vi "MegaAwesome_10_10_12a_JW.vi"() -> ()   [LabVIEW 2011]
uses:
  data/MegaAwesome_States.ctl
  <vilib>/Utility/inputDevices.llb/keyboardAcquire.vi
  <vilib>/Utility/file.llb/Read From Spreadsheet File (string).vi
  <vilib>/Utility/file.llb/Write To Spreadsheet File (string).vi
panel:
  out "Save Next?":bool
  out "Image Center X":i32
  in  "Disable Flag":bool
  out "Index":string
  in  "Slider Min":dbl=5.0
  in  "Slider Max":dbl=5.0
  out "Opj X Axis":string
  out "X Axis Display Type":string
  in  "Index-Sat":dbl=5.0
  in  "Index-Lin":dbl=5.0
  in  "IndexLog-Lin":dbl=5.0
  in  "IndexLog-Sat":dbl=5.0 caption="Num Pts"
  out "Lin Id-Log Used":dbl[](array[numeric])
  out "Lin-Vg Array-Log Used":dbl[](array[numeric])
  in  "New: Comments":string
  out "Save Array":string[][](array[string])
  out "Folder Index":i32 caption="Length"
  out "Sat Id-Used":dbl[](array[numeric])
  out "Sat Vg Array-Used":dbl[](array[numeric])
  out "Vg Array-Log-Used":dbl[](array[numeric])
  out "Sat Id-Log-Used":dbl[](array[numeric])
  out "Lin Id-Used":dbl[](array[numeric])
  out "Lin-Vg Array-Used":dbl[](array[numeric])
  out "Lin Vd":dbl
  out "Recorded Prop":T1
  out "Current State":T2
  in  "Main Tab Control":T3(tab)
  in  "Transfer File":path
  out "Transfer Folder":path
  in  "Transport\nFolder":path caption="Transport Folder"
  out "Transport\nFile":path caption="Transport File"
  in  "Image Folder":path
  out "Image File":path
  out "Fabrication Prop":T4
  out "Distances":i32[](array[numeric])
  in  "Zoom":i32(slide)=-3 scale=-5.0..5.0
  in  "Magnification":i32(ring) items=["5x", "10x", "20x", "50x", "80x"]
  in  "Undo Button":bool
  in  "Remove Button":bool
  in  "Transfer Plots":T5(tab)=enum."Saturation"
  in  "Lin-Trans Slider":dbl(slide) step=1.0 scale=-40.0..40.0 scale format="%#_1p"
  out "Sqrt-Lin":cluster{dbl[], dbl[]}[](graph)
  in  "Sat-Trans Slider":dbl(slide) step=1.0 scale=-40.0..40.0 scale format="%#_1p"
  out "Sqrt-Sat":cluster{dbl[], dbl[]}[](graph)
  out "Raw- Lin":cluster{dbl[], dbl[]}[](graph)
  out "Raw- Sat":cluster{dbl[], dbl[]}[](graph)
  in  "Log Plots":enum32{"Linear", "Saturation", "Transport"}(tab)=enum."Saturation"
  in  "Lin-Log Slider":dbl(slide) step=1.0 scale=-40.0..40.0 scale format="%#_1p"
  out "Lin-Log":cluster{dbl[], dbl[]}[](graph)
  in  "Sat-Log Slider":dbl(slide) step=1.0 scale=-40.0..40.0 scale format="%#_1p"
  out "Sat-Log":cluster{dbl[], dbl[]}[](graph)
  out "Transport":cluster{ext[], ext[]}[](graph)
  out "Transport Name:":string
  in  "Manual Controls":T6
  in  "File Controls":T7
  out "Date Recorded":string="Date Recorded" caption="Measured"
  out "Data Name:":string
  out "Image Name":string
  out "Date Created":string caption="Fabricated"
  in  "Comments:":string
  out "Rec: Length":dbl caption="Length" format="%#_3g"
  out "Rec: Width":dbl caption="Width" format="%#_4g"
  out "Rec: Dielectric (d)":dbl caption="Dielectric (d)" format="%#_3g"
  in  "New: Dielectric":dbl
  in  "New: Length":dbl
  in  "New: Width":dbl
  out "Rec: Temp":dbl caption="Sample Temp" format="%.1f"
  in  "New: Temp":dbl format="%.1f"
  out "Image Out":T8(plugin-control)
  in  "Num Pts":dbl=5.0
  in  "Num Pts Log":dbl=5.0 caption="Num Pts"
  out "Recorded Values Cluster":T9
  out "Calculated Values Cluster":T9 caption="Recorded Values Cluster"
  out "Re-Calculated Values Cluster":T9 caption="Recorded Values Cluster"
  in  "Independant Variable:":string(combo)="Length (um):"
  out "Image Preview":T8(plugin-control)
  out "Total Width":i32
  in  "Index Array":i32(ring) caption="Index" items=["4C", "4C", "4C", "4C", "4C", "4C", "4C", "4C", "4C", "4C", "4C", "4C", "4C", "4C", "4C", "4C", "4C", "4C", "4C", "4C", "4C", "4C", "4C", "4C", "4C", "4C", "4C", "4C", "4C", "4C", "4C", "4C", "4C", "4C", "4C", "4C", "4C", "4C", "4C"]
  in  "Room Temp":dbl=294.0 caption="Room Temp (K)"
  out "No Image\n File":path=path "\\\\acad1\\physics/Jurchescu-group/JW-PD/Mega Awesome/Image Not Found.png" caption="No Image File"
  out "Origin Project File":path=path "\\\\acad1\\physics/Jurchescu-group/JW-PD/Group Library/Origin Project Files/DeviceData_8_10_12a_JW.opj"
  out "No Transport\n File":path=path "\\\\acad1\\physics/Jurchescu-group/JW-PD/Mega Awesome/No Transport File.txt" caption="No Transport File"
  in  "Transport Style Controls":T10={"Transport Line Size"=1, "Transport Line Color"=16772608} {"Transport Line Size" items=["Extra Small", "Small", "Medium", "Large", "Extra Large"]}
  out "Application Directory":path
  # "1)  Select the Transfer File that you would like to analyze:"
  # "Transfer Location"
  # "2) What else would you like to view during your analysis?"
  # "Transport Location"
  # "Image Location"
  # "Recorded"
  # "Calculated"
  # "Re-Calculated"
  # "Manual"
  # "um"
  # "Slider\nDoesn't\nWork"
  # "V"
  # "V"
  # "Slider\nDoesn't\nWork"
  # "V"
  # "Default File Choices"
  # "Default Analysis Values"
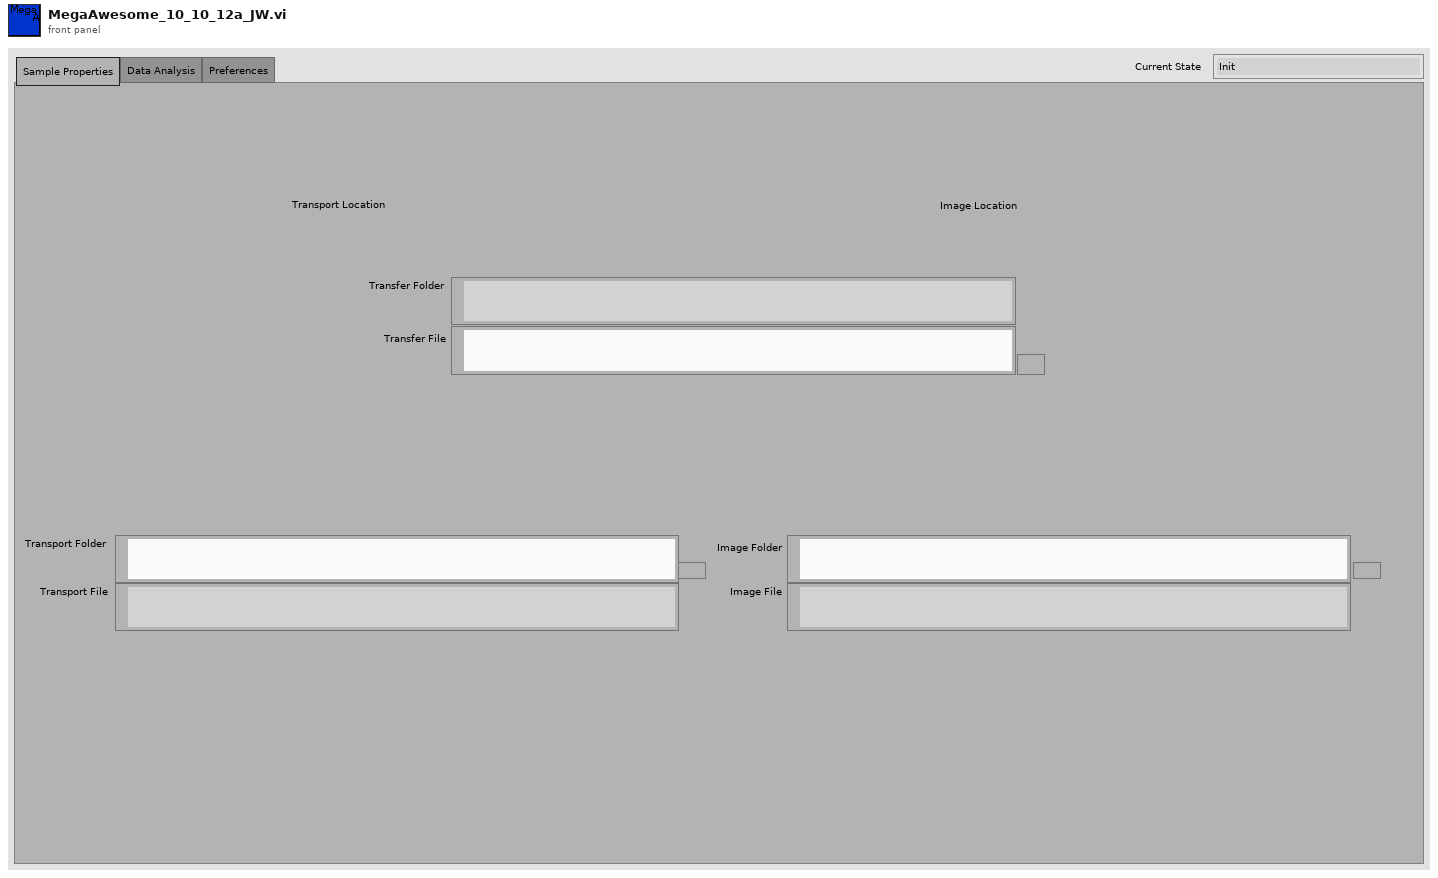
[diagram p1: front panel]
types:
  T1 = cluster{"Date Recorded":string, "Index":string, "Length":dbl, "Width":dbl, "Sample Temp":dbl}
  T2 = typedef "MegaAwesome_States.ctl" = enum16{"Init", "File Missing", "No Event", "Read Data", "Calculated Values", "Re-Calculated Values", "Next File", "Previous File", "Discard File", "Save", "Save Lines", "Export", "Exit"}
  T3 = enum32{"Sample Properties", "Data Analysis", "Preferences"}
  T4 = cluster{"Date Created":string, "Material":string, "Solvent":string, "Concentration":dbl, "Method":string, "Dielectric (nm)":dbl, "Treatment":string, "Comments":string}
  T5 = enum32{"Linear", "Saturation", "Raw-Linear", "Raw-Saturation"}
  T6 = cluster{"Manual-Temp":bool, "Manual-Width":bool, "Manuel-Length":bool, "Manuel-Dielectric":bool, "Manual Comments":bool}
  T7 = cluster{"Previous File":bool, "Discard ":bool, "Save Lines":bool, "Close":bool, "Next File ":bool, "Save":bool, "Save Next":bool, "Export":bool}
  T8 = typedef "IMAQ Image.ctl" = refnum<image>
  T9 = cluster{"Mobility-Sat":dbl, "Moblitity-Lin":dbl, "On/Off":dbl, "Off Current":dbl, "Vt-Sat":dbl, "STS":dbl, "Trap Density-VT":dbl, "Trap Density-STS":dbl}
  T10 = cluster{"Transport Line Size":u16, "Transport Line Color":u32}
  T11 = typedef "LVBoundsTypeDef.ctl" = cluster{"Width":u32, "Height":u32}
  T12 = enum16{"0", "1", "2", "3", "4", "5", "6", "7", "8", "9", "A", "B", "C", "D", "E", "F", "G", "H", "I", "J", "K", "L", "M", "N", "O", "P", "Q", "R", "S", "T", "U", "V", "W", "X", "Y", "Z", "F1", "F2", "F3", "F4", "F5", "F6", "F7", "F8", "F9", "F10", "F11", "F12", "F13", "F14", "F15", "ADD", "BACK", "BACKSLASH", "CAPITAL", "COMMA", "DECIMAL", "DELETE", "DIVIDE", "DOWN", "END", "EQUALS", "ESCAPE", "GRAVE (`)", "HOME", "INSERT", "LBRACKET", "LCONTROL", "LEFT", "L ALT", "LSHIFT", "LWIN", "MINUS", "MULTIPLY", "NEXT", "NUMLOCK", "NUMPAD_0", "NUMPAD_1", "NUMPAD_2", "NUMPAD_3", "NUMPAD_4", "NUMPAD_5", "NUMPAD_6", "NUMPAD_7", "NUMPAD_8", "NUMPAD_9", "PAUSE", "PERIOD", "PRIOR (PG UP)", "RBRACKET", "RCONTROL", "RETURN", "RIGHT", "R ALT", "RSHIFT", "RWIN", "SCROLL", "SEMICOLON", "SLASH", "SPACE", "SUBTRACT", "TAB", "UP", "ENTER (num pad)", "' (quote)"}[]
  T13 = enum16{"0", "1", "2", "3", "4", "5", "6", "7", "8", "9", "A", "B", "C", "D", "E", "F", "G", "H", "I", "J", "K", "L", "M", "N", "O", "P", "Q", "R", "S", "T", "U", "V", "W", "X", "Y", "Z", "F1", "F2", "F3", "F4", "F5", "F6", "F7", "F8", "F9", "F10", "F11", "F12", "F13", "F14", "F15", "ADD", "BACK", "BACKSLASH", "CAPITAL", "COMMA", "DECIMAL", "DELETE", "DIVIDE", "DOWN", "END", "EQUALS", "ESCAPE", "GRAVE (`)", "HOME", "INSERT", "LBRACKET", "LCONTROL", "LEFT", "L ALT", "LSHIFT", "LWIN", "MINUS", "MULTIPLY", "NEXT", "NUMLOCK", "NUMPAD_0", "NUMPAD_1", "NUMPAD_2", "NUMPAD_3", "NUMPAD_4", "NUMPAD_5", "NUMPAD_6", "NUMPAD_7", "NUMPAD_8", "NUMPAD_9", "PAUSE", "PERIOD", "PRIOR (PG UP)", "RBRACKET", "RCONTROL", "RETURN", "RIGHT", "R ALT", "RSHIFT", "RWIN", "SCROLL", "SEMICOLON", "SLASH", "SPACE", "SUBTRACT", "TAB", "UP", "ENTER (num pad)", "' (quote)"}
  T14 = typedef "ROI Descriptor" = cluster{"Global Rectangle":i32[], "Contours":cluster{"ID":enum32{"External", "Internal"}, "Type":u32, "Coordinates":i32[]}[]}
  T15 = cluster{string, dbl, bool, bool, bool, bool, bool, bool, i32}
  T16 = cluster{i32, cluster{string, dbl, bool, bool, bool, bool, bool, bool, i32}, i32, i32}
  T17 = cluster{"Global Rectangle":i32[], "Contours":cluster{"Contour Type":u32, "ROI Type":u32, "Points":i32[]}[]}
  T18 = cluster{"Contour Type":u32, "ROI Type":u32, "Points":i32[]}[]
  T19 = cluster{"[0]":cluster{dbl[], dbl[]}, "[1]":cluster{dbl[], dbl[]}, "[2]":cluster{dbl[], dbl[]}, "[3]":cluster{dbl[], dbl[]}, "[4]":cluster{dbl[], dbl[]}, "[5]":cluster{dbl[], dbl[]}, "[6]":cluster{dbl[], dbl[]}, "[7]":cluster{dbl[], dbl[]}, "[8]":cluster{dbl[], dbl[]}}
  T20 = cluster{i32[], cluster{"Contour Type":u32, "ROI Type":u32, "Points":i32[]}[]}
  T21 = cluster{"Contour Type":u32, "ROI Type":u32, "Points":i32[]}
  T22 = cluster{"Points[0]":i32, "Points[1]":i32, "Points[2]":i32, "Points[3]":i32, "Points[4]":i32, "Points[5]":i32, "Points[6]":i32, "Points[7]":i32, "Points[8]":i32}
  T23 = cluster{"Sat Vg Used":dbl[], "Sat Sqrt(Id) Used ":dbl[], "Lin Vg Used":dbl[], "Lin Sqrt(Id) Used":dbl[], "Index-Lin":dbl, "Index-Sat":dbl}
  T24 = cluster{"Raw Sat":cluster{dbl[], dbl[]}[], "Sqrt Sat":cluster{dbl[], dbl[]}[], "Log Sat":cluster{dbl[], dbl[]}[], "Raw Lin":cluster{dbl[], dbl[]}[], "Sqrt Lin":cluster{dbl[], dbl[]}[], "Log Lin":cluster{dbl[], dbl[]}[]}
  T25 = cluster{"Mobility-Sat":dbl, "Vt-Sat":dbl, "Mobility-Lin":dbl, "Vt-Lin":dbl, "Off I-Sat":dbl, "On/Off I-Sat":dbl}
  T26 = cluster{"Sat Vg Used":dbl[], "Sat Log(Id) Used":dbl[], "Lin Vg Used":dbl[], "Lin Log(Id) Used":dbl[], "STS Index-Sat":dbl, "STS Index-Lin":dbl}
  T27 = cluster{"Independant  Variable Indicator":string, "Parameter String Indicator":string}
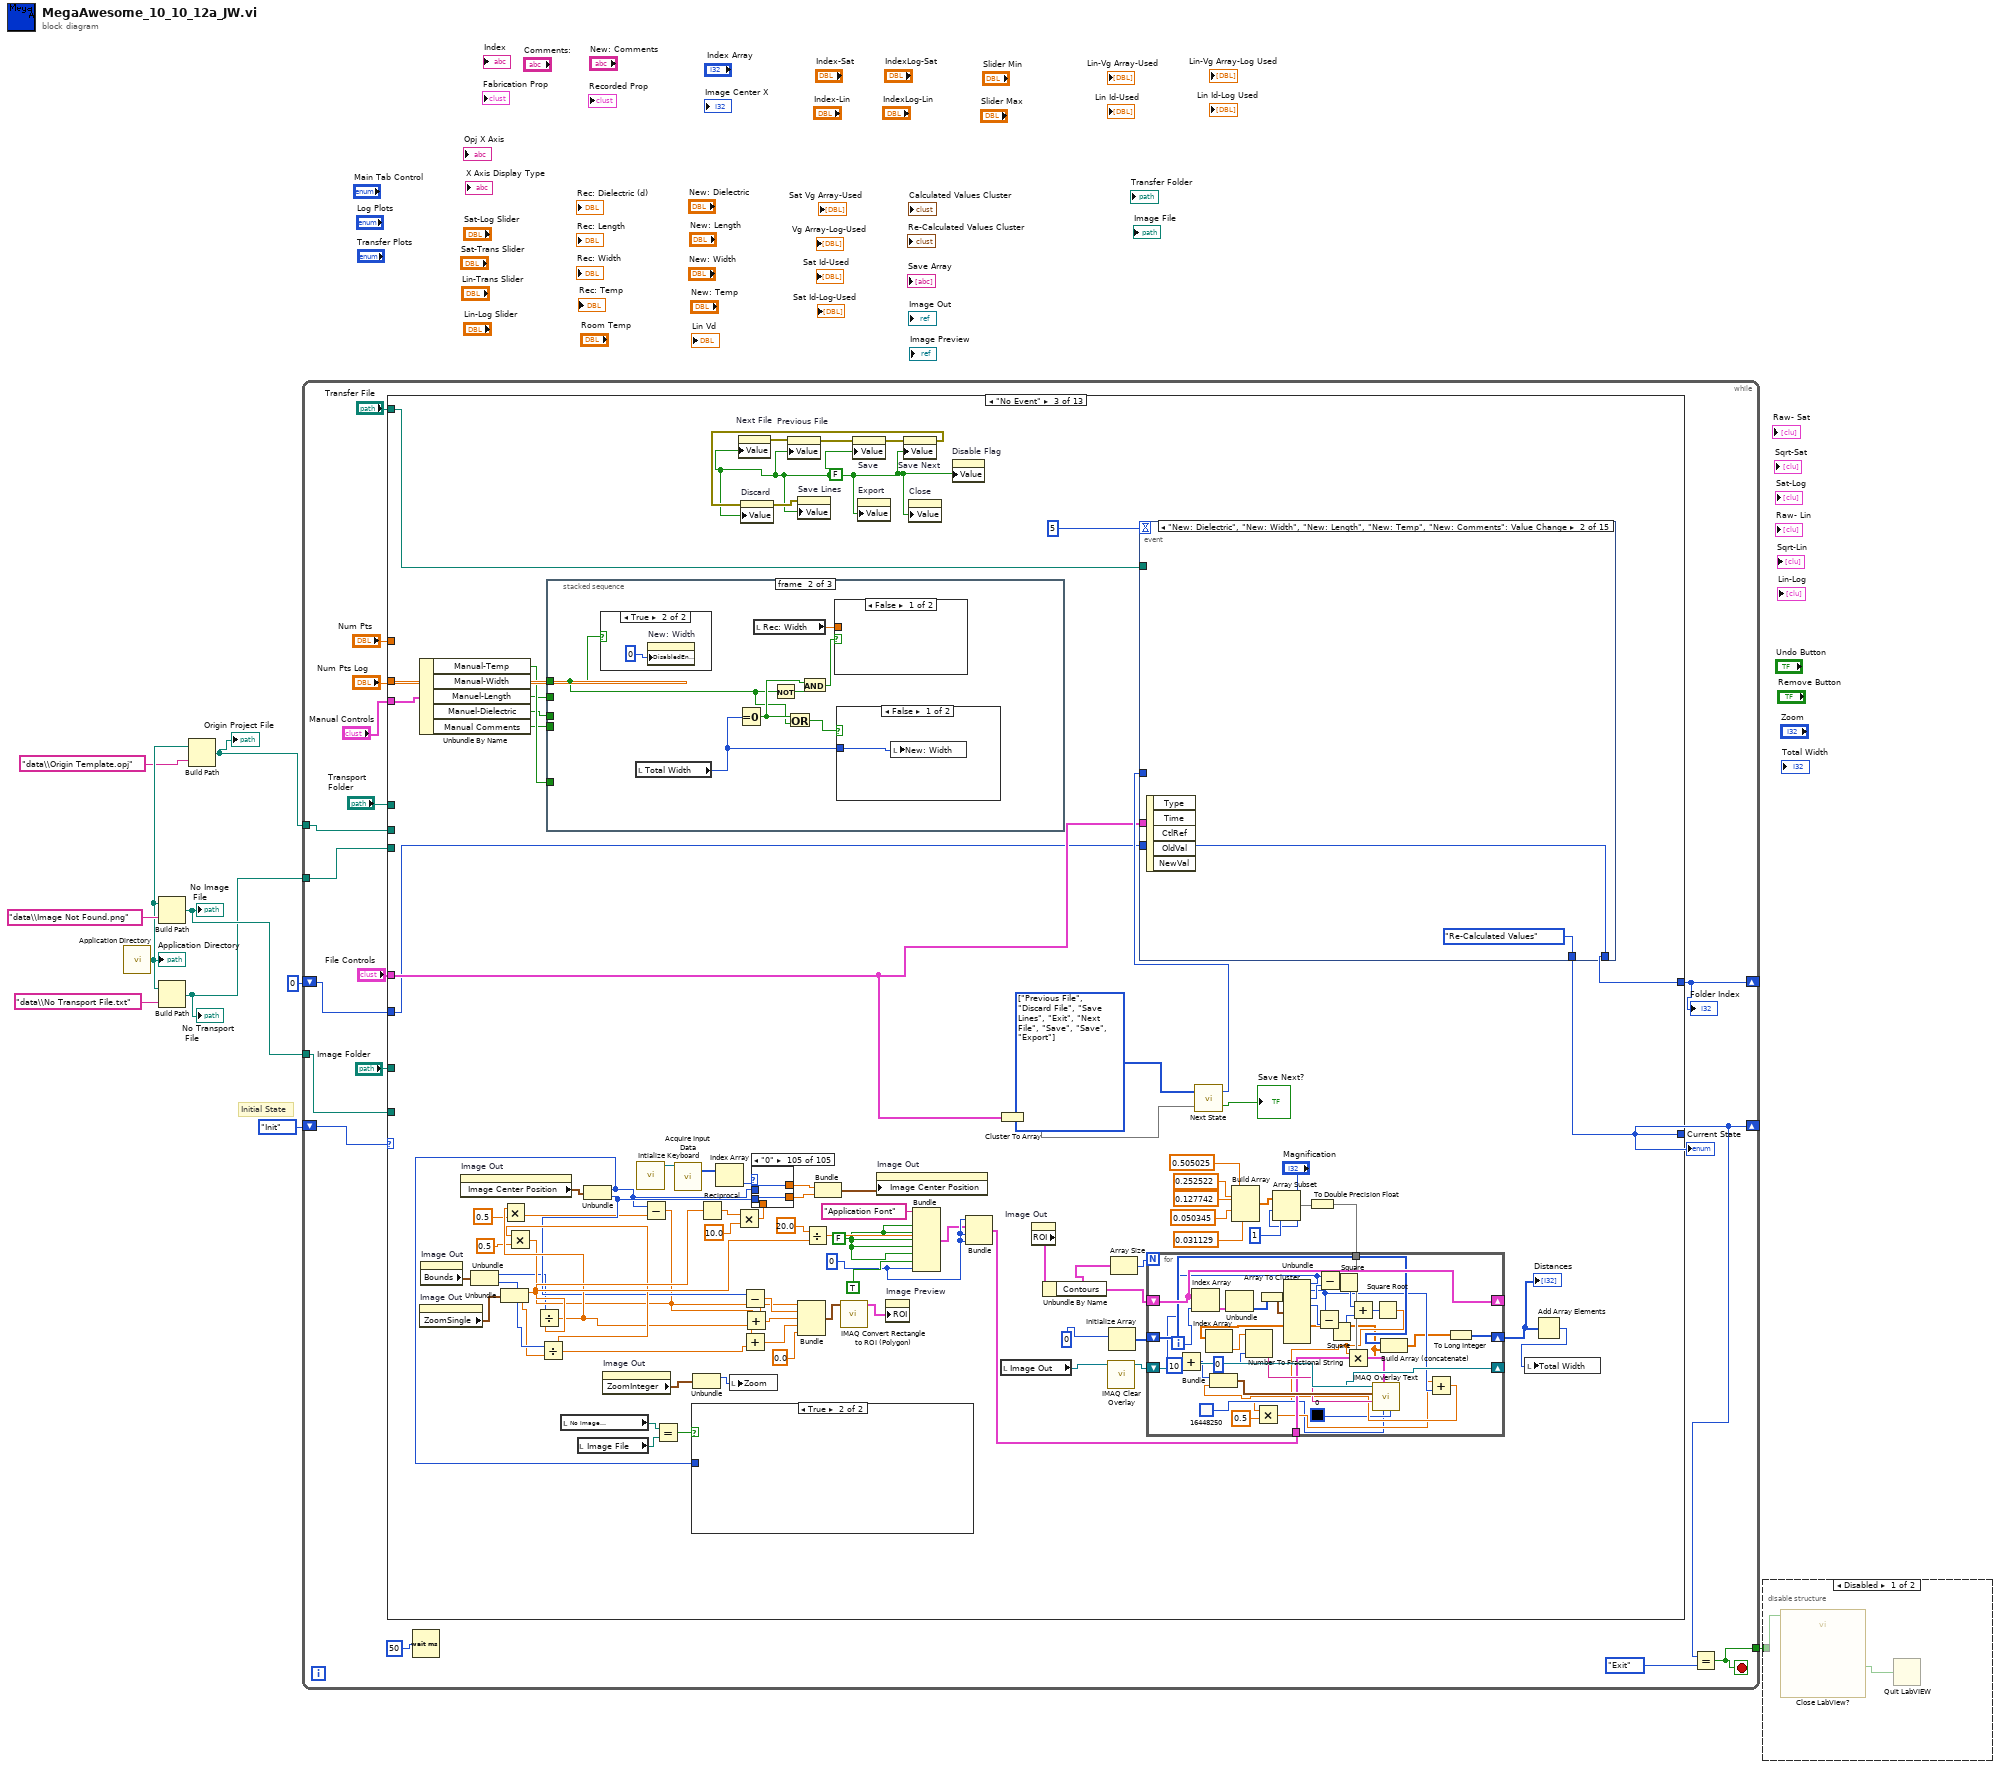
[diagram p0: block diagram]
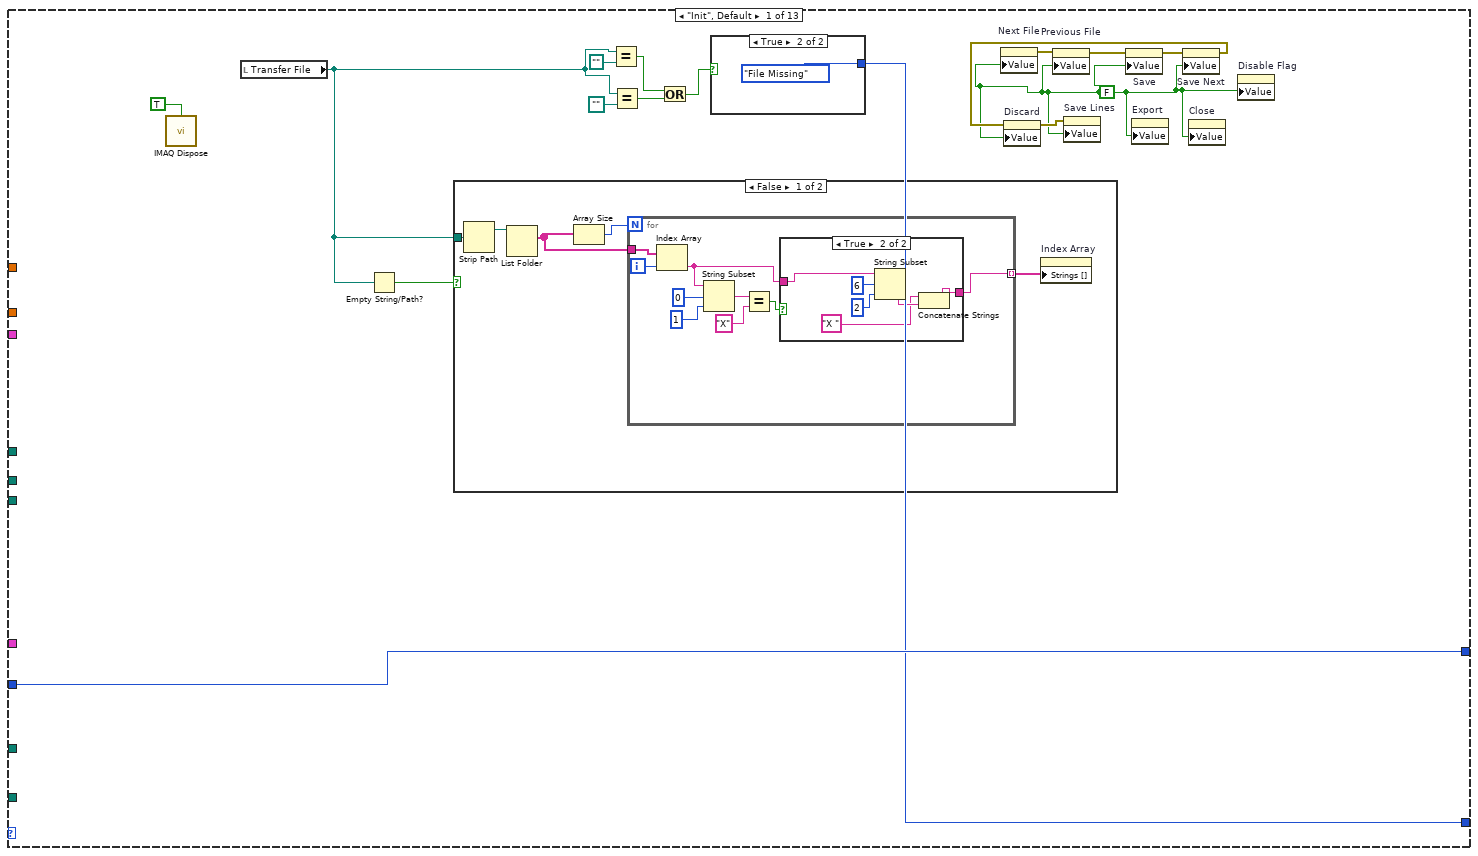
[diagram p3: hidden frame]
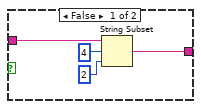
[diagram p4: hidden frame]
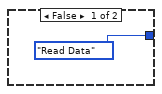
[diagram p6: hidden frame]
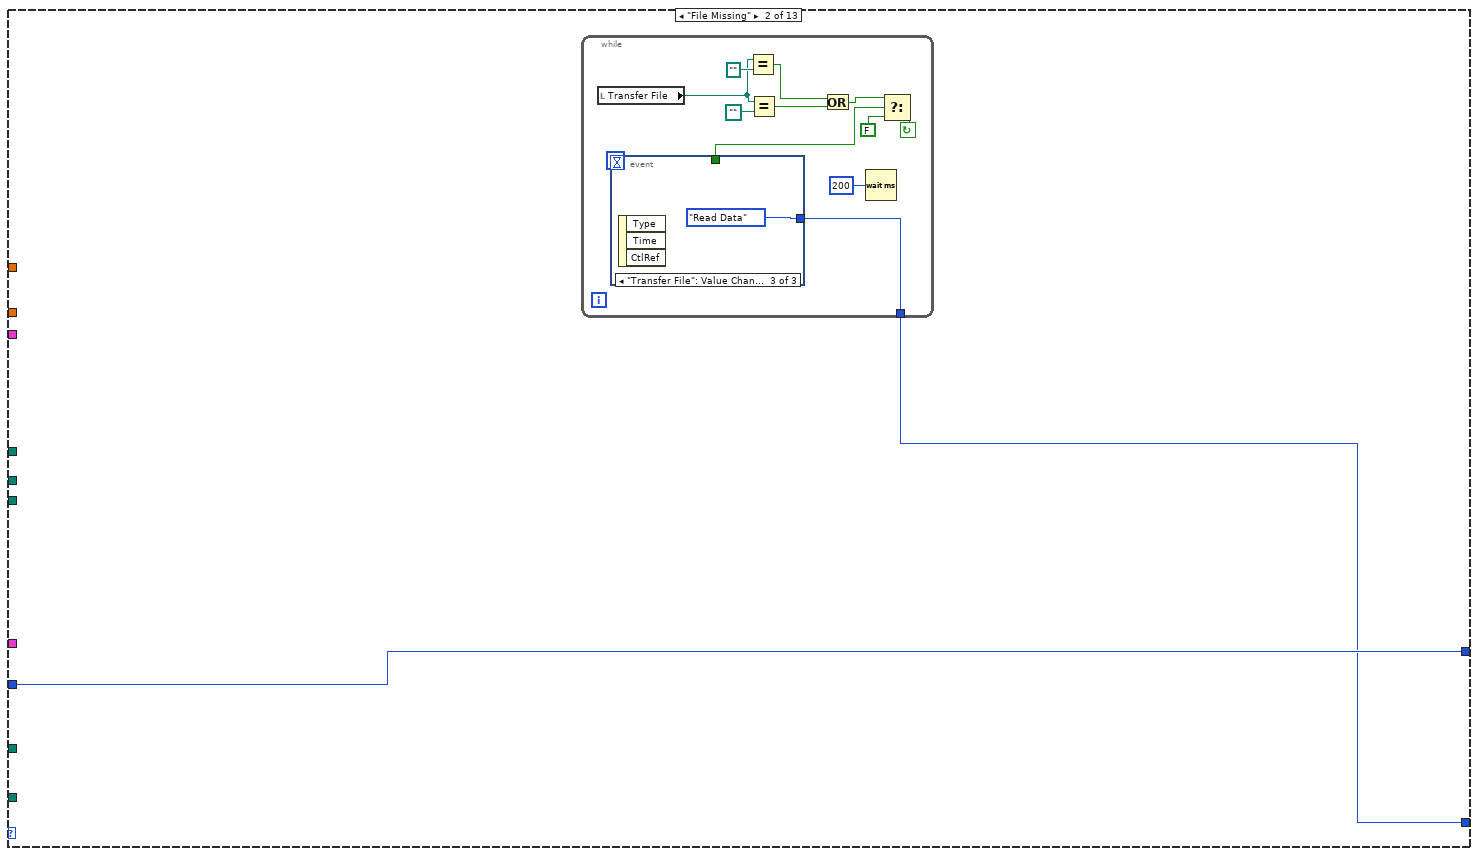
[diagram p7: hidden frame]
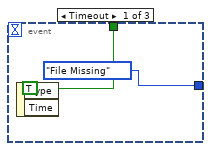
[diagram p8: hidden frame]
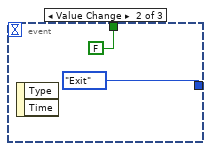
[diagram p9: hidden frame]
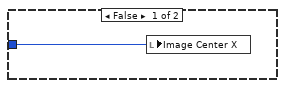
[diagram p10: hidden frame]
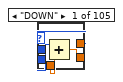
[diagram p11: hidden frame]
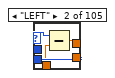
[diagram p12: hidden frame]
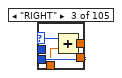
[diagram p13: hidden frame]
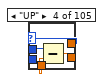
[diagram p14: hidden frame]
diagram:
  # "Initial State"
  n1 = call <vilib>:"Application Directory.vi"() -> ("Application Directory"=w3:path)
  "Application Directory" <- w3
  n2 = Build Path(base path=w3, name or relative path="data\\Image Not Found.png") -> (appended path=w6:path)
  "No Image\n File" <- w6
  n3 = Build Path(base path=w3, name or relative path="data\\No Transport File.txt") -> (appended path=w5:path)
  "No Transport\n File" <- w5
  n4 = Build Path(base path=w3, name or relative path="data\\Origin Template.opj") -> (appended path=w4:path)
  "Origin Project File" <- w4
  n5 = while {
    shift-right: [w11] -> _
    shift-left: MegaAwesome_States."Init" -> [w13]
    shift-right: [w21] -> _
    shift-left: 0 -> [w22]
    tunnel: w6 -> [w18]
    tunnel: w5 -> [w16]
    tunnel: w4 -> [w15]
    tunnel: [w14] -> w1
    stop <- w14 stop-if-true
    n6 = case shown="\"No Event\"" w13 {
      tunnel: [w28 w70 w164 MegaAwesome_States."Calculated Values" MegaAwesome_States."Re-Calculated Values" MegaAwesome_States."No Event" MegaAwesome_States."Read Data" MegaAwesome_States."Read Data" MegaAwesome_States."Init" w815 MegaAwesome_States."Exit" MegaAwesome_States."No Event" MegaAwesome_States."No Event"] -> w11
      tunnel: "Transfer File" -> [_ _ w156 w614 w662 _ w763 w774 w801 w820 _ _ _]
      tunnel: "Num Pts" -> [_ _ _ _ w697 _ _ _ _ _ _ _ _]
      tunnel: "Num Pts Log" -> [_ _ _ _ w696 _ _ _ _ _ _ _ _]
      tunnel: "Image Folder" -> [_ _ _ _ w693 _ _ _ _ _ _ w1350 _]
      tunnel: w18 -> [_ _ _ _ w692 _ _ _ _ _ _ _ _]
      tunnel: [w38 w71 w157 w619 w691 w723 w749 w772 w797 w821 w1336 w1360 w1366] -> w21
      tunnel: w22 -> [w38 w71 w89 w617 w691 w723 w750 w773 _ w821 w1336 w1360 w1366]
      tunnel: "Manual Controls" -> [_ _ w166 _ _ _ _ _ _ w819 _ _ _]
      tunnel: "File Controls" -> [_ _ w154 _ _ _ _ _ _ _ _ _ _]
      tunnel: "Transport\nFolder" -> [_ _ _ _ w658 _ _ _ _ _ _ _ _]
      tunnel: w16 -> [_ _ _ _ w657 _ _ _ _ _ _ _ _]
      tunnel: w15 -> [_ _ _ _ _ _ _ _ _ _ _ _ w1365]
      frame "Init", Default {
        w29 = FALSE
        n7 = call "IMAQ Dispose"("All Images? (No)"=TRUE) -> ()  [unwired: 5 in, 1 out]
        n8 = local read "Transfer File"() -> (w36:path)
        n9 = Empty String/Path?(string/path=w36) -> (empty?=w37:bool)
        n10 = case shown="False" w37 {
          tunnel: w36 -> [w45 _]
          frame False {
            n11 = Strip Path(path=w45) -> (stripped path=w47:path)  [unwired: 1 out]
            n12 = List Folder(path=w47) -> (filenames=w46:string[])  [unwired: 3 in, 3 out]
            n13 = Array Size(array=w46) -> (size(s)=w48:i32)
            n14 = for {
              N: w48 -> [_]
              tunnel: w46 -> [w57]
              tunnel: [w55] -> w44 mode=indexing
              i -> [w56]
              n15 = Index Array(array=w57, index=w56) -> (element=w54:string)
              n16 = String Subset(string=w54, offset (0)=0, length (rest)=1) -> (substring=w51:string)
              n17 = Equal?(x=w51, y="X") -> (x = y?=w50:bool)
              n18 = case shown="True" w50 {
                tunnel: w54 -> [w61 w65]
                tunnel: [w58 w64] -> w55
                frame False {
                  n19 = String Subset(string=w61, offset (0)=4, length (rest)=2) -> (substring=w58:string)
                }
                frame True {
                  n20 = String Subset(string=w65, offset (0)=6, length (rest)=2) -> (substring=w63:string)
                  n21 = Concatenate Strings("X ", w63) -> (w64:string)
                }
              }
            }
            n22 = property on="Index Array" class="Ring (strict)"("Strings []"=w44) -> ()  [unwired: 2 in, 2 out]
          }
          frame True {
          }
        }
        n23 = Equal?(x=w36, y=path "") -> (x = y?=w41:bool)
        n24 = Equal?(x=w36, y=path "") -> (x = y?=w40:bool)
        n25 = Or(x=w41, y=w40) -> (x .or. y?=w43:bool)
        n26 = case shown="True" w43 {
          tunnel: [MegaAwesome_States."Read Data" MegaAwesome_States."File Missing"] -> w28
          frame False {
          }
          frame True {
          }
        }
        n27 = property on="Next File" class="Bool (strict)"("Value"=w29) -> (error out=w34:errorcluster)  [unwired: 2 in, 1 out]
        n28 = property on="Previous File" class="Bool (strict)"(error in=w34, "Value"=w29) -> (error out=w33:errorcluster)  [unwired: 1 in, 1 out]
        n29 = property on="Save" class="Bool (strict)"(error in=w33, "Value"=w29) -> (error out=w32:errorcluster)  [unwired: 1 in, 1 out]
        n30 = property on="Export" class="Bool (strict)"("Value"=w29) -> ()  [unwired: 2 in, 2 out]
        n31 = property on="Save Next" class="Bool (strict)"(error in=w32, "Value"=w29) -> (error out=w31:errorcluster)  [unwired: 1 in, 1 out]
        n32 = property on="Discard" class="Bool (strict)"(error in=w31, "Value"=w29) -> (error out=w30:errorcluster)  [unwired: 1 in, 1 out]
        n33 = property on="Save Lines" class="Bool (strict)"(error in=w30, "Value"=w29) -> ()  [unwired: 1 in, 2 out]
        n34 = property on="Close" class="Bool (strict)"("Value"=w29) -> ()  [unwired: 2 in, 2 out]
        n35 = property on="Disable Flag" class="Bool (strict)"("Value"=w29) -> ()  [unwired: 2 in, 2 out]
      }
      frame "File Missing" {
        n36 = while {
          tunnel: [w78] -> w70
          stop <- w74 continue-if-true
          n37 = local read "Transfer File"() -> (w79:path)
          n38 = event shown="[2] \"Transfer File\": Value Change" {
            selector: _ -> [_ _ _]
            dyn-events: _ -> [_ _ _]
            timeout: 10 -> [_ _ _]
            tunnel: [MegaAwesome_States."File Missing" MegaAwesome_States."Exit" MegaAwesome_States."Read Data"] -> w78
            tunnel: [TRUE FALSE _] -> w77
            event Timeout {
              n39 = event-data() -> ()  [unwired: 1 in, 2 out]
            }
            event "File Controls.Close": Value Change {
              n40 = event-data() -> ()  [unwired: 1 in, 2 out]
            }
            event "Transfer File": Value Change {
              n41 = event-data() -> ()  [unwired: 1 in, 3 out]
            }
          }
          n42 = Equal?(x=w79, y=path "") -> (x = y?=w81:bool)
          n43 = Equal?(x=w79, y=path "") -> (x = y?=w82:bool)
          n44 = Or(x=w81, y=w82) -> (x .or. y?=w76:bool)
          n45 = Wait (ms)(milliseconds to wait=u32 200) -> ()  [unwired: 1 out]
          n46 = Select(t=w76, s=w77, f=FALSE) -> (s? t:f=w74:bool)
        }
      }
      frame "No Event" {
        w145 = FALSE
        w147 = 0
        w155 = FALSE
        w173 = T2[] [enum."Previous File", enum."Discard File", enum."Save Lines", enum."Exit", enum."Next File", enum."Save", enum."Save", enum."Export"] items=["Init", "File Missing", "No Event", "Read Data", "Calculated Values", "Re-Calculated Values", "Next File", "Previous File", "Discard File", "Save", "Save Lines", "Export", "Exit"]
        n47 = Unbundle By Name(w166) -> ("Manual-Temp"=w171:bool, "Manual-Width"=w170:bool, "Manuel-Length"=w169:bool, "Manuel-Dielectric"=w168:bool, "Manual Comments"=w167:bool)
        n48 = property on="Image Out" class="ImageControl"() -> ("ZoomSingle"=w131:cluster{"X":sgl, "Y":sgl})  [unwired: 2 in, 2 out]
        n49 = property on="Image Out" class="ImageControl"() -> ("Bounds"=w130:T11)  [unwired: 2 in, 2 out]
        n50 = property on="Image Out" class="ImageControl"() -> ("Image Center Position"=w124:cluster{"X":u32, "Y":u32})  [unwired: 2 in, 2 out]
        n51 = Unbundle(w130) -> ("Width"=w133:u32, "Height"=w134:u32)
        n52 = Unbundle(w131) -> ("X"=w151:sgl, "Y"=w132:sgl)
        n53 = Divide(x=w133, y=w151) -> (x/y=w142:sgl)
        n54 = Multiply(x=w142, y=0.5) -> (x*y=w137:dbl)
        n55 = Divide(x=w134, y=w132) -> (x/y=w143:sgl)
        n56 = Multiply(x=w143, y=0.5) -> (x*y=w138:dbl)
        n57 = stacked-sequence {
          tunnel: w171 -> [w573 _ _]
          tunnel: w170 -> [_ w582 _]
          tunnel: w169 -> [_ _ w598]
          tunnel: w168 -> [_ _ w595]
          tunnel: w167 -> [_ _ w594]
          frame #0 {
            n58 = local read "Rec: Temp"() -> (w572:dbl)
            n59 = case shown="False" w573 {
              tunnel: w572 -> [w578 _]
              frame False {
                n60 = local read "Rec: Temp"() -> (w576:dbl)
                n61 = property on="New: Temp" class="DigNum (strict)"("DisabledEnum"=1) -> ()  [unwired: 2 in, 2 out]
                n62 = Equal To 0?(x=w576) -> (x = 0?=w577:bool)
                n63 = local write "New: Temp"(w578) -> ()
                n64 = case shown="True" w577 {
                  tunnel: [w579 w580] -> w574
                  tunnel: w576 -> [w579 _]
                  frame False {
                  }
                  frame True {
                    n65 = local read "Room Temp"() -> (w580:dbl)
                  }
                }
                n66 = local write "Rec: Temp"(w574) -> ()
                n67 = local write "New: Temp"(w574) -> ()
              }
              frame True {
                n68 = property on="New: Temp" class="DigNum (strict)"("DisabledEnum"=0) -> ()  [unwired: 2 in, 2 out]
              }
            }
          }
          frame #1 {
            n69 = case shown="True" w582 {
              frame False {
                n70 = property on="New: Width" class="DigNum (strict)"("DisabledEnum"=1) -> ()  [unwired: 2 in, 2 out]
              }
              frame True {
                n71 = property on="New: Width" class="DigNum (strict)"("DisabledEnum"=0) -> ()  [unwired: 2 in, 2 out]
              }
            }
            n72 = local read "Total Width"() -> (w588:i32)
            n73 = Equal To 0?(x=w588) -> (x = 0?=w585:bool)
            n74 = local read "Rec: Width"() -> (w586:dbl)
            n75 = Not(x=w582) -> (.not. x?=w584:bool)
            n76 = Or(x=w585, y=w582) -> (x .or. y?=w587:bool)
            n77 = And(x=w585, y=w584) -> (x .and. y?=w583:bool)
            n78 = case shown="False" w583 {
              tunnel: w586 -> [_ w591]
              frame False {
              }
              frame True {
                n79 = local write "New: Width"(w591) -> ()
              }
            }
            n80 = case shown="False" w587 {
              tunnel: w588 -> [w592 _]
              frame False {
                n81 = local write "New: Width"(w592) -> ()
              }
              frame True {
                n82 = property on="New: Width" class="DigNum (strict)"("DisabledEnum"=0) -> ()  [unwired: 2 in, 2 out]
              }
            }
          }
          frame #2 {
            n83 = local read "Rec: Length"() -> (w599:dbl)
            n84 = case shown="False" w598 {
              tunnel: w599 -> [w607 _]
              frame False {
                n85 = local write "New: Length"(w607) -> ()
                n86 = property on="New: Length" class="DigNum (strict)"("DisabledEnum"=u8 1) -> ()  [unwired: 2 in, 2 out]
              }
              frame True {
                n87 = property on="New: Length" class="DigNum (strict)"("DisabledEnum"=0) -> ()  [unwired: 2 in, 2 out]
              }
            }
            n88 = local read "Comments:"() -> (w596:string)
            n89 = local read "Rec: Dielectric (d)"() -> (w597:dbl)
            n90 = case shown="False" w594 {
              tunnel: w596 -> [w601 _]
              frame False {
                n91 = local write "New: Comments"(w601) -> ()
                n92 = property on="New: Comments" class="Str"("DisabledEnum"=1) -> ()  [unwired: 2 in, 2 out]
              }
              frame True {
                n93 = property on="New: Comments" class="Str"("DisabledEnum"=0) -> ()  [unwired: 2 in, 2 out]
              }
            }
            n94 = case shown="True" w595 {
              tunnel: w597 -> [w604 _]
              frame False {
                n95 = local write "New: Dielectric"(w604) -> ()
                n96 = property on="New: Dielectric" class="DigNum (strict)"("DisabledEnum"=1) -> ()  [unwired: 2 in, 2 out]
              }
              frame True {
                n97 = property on="New: Dielectric" class="DigNum (strict)"("DisabledEnum"=0) -> ()  [unwired: 2 in, 2 out]
              }
            }
          }
        }
        n98 = local read "No Image\n File"() -> (w95:path)
        n99 = local read "Image File"() -> (w94:path)
        n100 = Unbundle(w124) -> ("X"=w96:u32, "Y"=w141:u32)
        n101 = property on="Image Out" class="ImageControl"() -> ("ZoomInteger"=w99:cluster{"X":i32, "Y":i32})  [unwired: 2 in, 2 out]
        n102 = call <vilib>:"Intialize Keyboard.vi"() -> ("device ID"=w121:refnum<k1>)  [unwired: 10 in, 1 out]
        n103 = Subtract(x=w96, y=w137) -> (x-y=w139:dbl)
        n104 = Equal?(x=w95, y=w94) -> (x = y?=w93:bool)
        n105 = call-poly <vilib>:"Acquire Input Data.vi"("device ID"=w121) -> ("keys pressed"=w122:T12)  [unwired: 16 in, 2 out]
        n106 = case shown="True" w93 {
          tunnel: w96 -> [w174 _]
          frame False {
            n107 = local write "Image Center X"(w174) -> ()
          }
          frame True {
          }
        }
        n108 = Unbundle(w99) -> ("X"=w98:i32)  [unwired: 1 out]
        n109 = Reciprocal(x=w151) -> (1/x=w152:sgl)
        n110 = Index Array(array=w122) -> (element=w118:T13)  [unwired: 1 in]
        n111 = local write "Zoom"(w98) -> ()
        n112 = Multiply(x=w152, y=sgl 10.0) -> (x*y=w150:sgl)
        n113 = property on="Next File" class="Bool (strict)"("Value"=w155) -> (error out=w162:errorcluster)  [unwired: 2 in, 1 out]
        n114 = Subtract(x=w141, y=w138) -> (x-y=w140:dbl)
        n115 = Add(x=w140, y=w143) -> (x+y=w126:dbl)
        n116 = Add(x=w139, y=w142) -> (x+y=w125:dbl)
        n117 = case shown="\"0\"" w118 {
          tunnel: w96 -> [w210 w216 w220 w222 w226 w228 w230 w232 w234 w236 w238 w240 w242 w244 w246 w248 w250 w252 w254 w256 w258 w260 w262 w264 w266 w268 w270 w272 w274 w276 w278 w280 w282 w284 w286 w288 w290 w292 w294 w296 w298 w300 w302 w304 w306 w308 w310 w312 w314 w316 w318 w320 w322 w324 w326 w328 w330 w332 w334 w336 w338 w340 w342 w344 w346 w348 w350 w352 w354 w356 w358 w360 w362 w364 w366 w368 w370 w372 w374 w376 w378 w380 w382 w384 w386 w388 w390 w392 w394 w396 w398 w400 w402 w404 w406 w408 w410 w412 w414 w416 w418 w420 w422 w424 w426]
          tunnel: [w210 w215 w219 w222 w226 w228 w230 w232 w234 w236 w238 w240 w242 w244 w246 w248 w250 w252 w254 w256 w258 w260 w262 w264 w266 w268 w270 w272 w274 w276 w278 w280 w282 w284 w286 w288 w290 w292 w294 w296 w298 w300 w302 w304 w306 w308 w310 w312 w314 w316 w318 w320 w322 w324 w326 w328 w330 w332 w334 w336 w338 w340 w342 w344 w346 w348 w350 w352 w354 w356 w358 w360 w362 w364 w366 w368 w370 w372 w374 w376 w378 w380 w382 w384 w386 w388 w390 w392 w394 w396 w398 w400 w402 w404 w406 w408 w410 w412 w414 w416 w418 w420 w422 w424 w426] -> w119
          tunnel: w141 -> [w212 w214 w218 w224 w225 w227 w229 w231 w233 w235 w237 w239 w241 w243 w245 w247 w249 w251 w253 w255 w257 w259 w261 w263 w265 w267 w269 w271 w273 w275 w277 w279 w281 w283 w285 w287 w289 w291 w293 w295 w297 w299 w301 w303 w305 w307 w309 w311 w313 w315 w317 w319 w321 w323 w325 w327 w329 w331 w333 w335 w337 w339 w341 w343 w345 w347 w349 w351 w353 w355 w357 w359 w361 w363 w365 w367 w369 w371 w373 w375 w377 w379 w381 w383 w385 w387 w389 w391 w393 w395 w397 w399 w401 w403 w405 w407 w409 w411 w413 w415 w417 w419 w421 w423 w425]
          tunnel: [w211 w214 w218 w223 w225 w227 w229 w231 w233 w235 w237 w239 w241 w243 w245 w247 w249 w251 w253 w255 w257 w259 w261 w263 w265 w267 w269 w271 w273 w275 w277 w279 w281 w283 w285 w287 w289 w291 w293 w295 w297 w299 w301 w303 w305 w307 w309 w311 w313 w315 w317 w319 w321 w323 w325 w327 w329 w331 w333 w335 w337 w339 w341 w343 w345 w347 w349 w351 w353 w355 w357 w359 w361 w363 w365 w367 w369 w371 w373 w375 w377 w379 w381 w383 w385 w387 w389 w391 w393 w395 w397 w399 w401 w403 w405 w407 w409 w411 w413 w415 w417 w419 w421 w423 w425] -> w120
          tunnel: w150 -> [w209 w213 w217 w221 _ _ _ _ _ _ _ _ _ _ _ _ _ _ _ _ _ _ _ _ _ _ _ _ _ _ _ _ _ _ _ _ _ _ _ _ _ _ _ _ _ _ _ _ _ _ _ _ _ _ _ _ _ _ _ _ _ _ _ _ _ _ _ _ _ _ _ _ _ _ _ _ _ _ _ _ _ _ _ _ _ _ _ _ _ _ _ _ _ _ _ _ _ _ _ _ _ _ _ _ _]
          frame "DOWN" {
            n118 = Add(x=w212, y=w209) -> (x+y=w211:sgl)
          }
          frame "LEFT" {
            n119 = Subtract(x=w216, y=w213) -> (x-y=w215:sgl)
          }
          frame "RIGHT" {
            n120 = Add(x=w220, y=w217) -> (x+y=w219:sgl)
          }
          frame "UP" {
            n121 = Subtract(x=w224, y=w221) -> (x-y=w223:sgl)
          }
          frame "ENTER (num pad)" {
          }
          frame "' (quote)" {
          }
          frame "END" {
          }
          frame "EQUALS" {
          }
          frame "ESCAPE" {
          }
          frame "GRAVE (`)" {
          }
          frame "HOME" {
          }
          frame "INSERT" {
          }
          frame "LBRACKET" {
          }
          frame "LCONTROL" {
          }
          frame "L ALT" {
          }
          frame "LSHIFT" {
          }
          frame "LWIN" {
          }
          frame "MINUS" {
          }
          frame "MULTIPLY" {
          }
          frame "NEXT" {
          }
          frame "NUMLOCK" {
          }
          frame "NUMPAD_0" {
          }
          frame "NUMPAD_1" {
          }
          frame "NUMPAD_2" {
          }
          frame "NUMPAD_3" {
          }
          frame "NUMPAD_4" {
          }
          frame "NUMPAD_5" {
          }
          frame "NUMPAD_6" {
          }
          frame "NUMPAD_7" {
          }
          frame "NUMPAD_8" {
          }
          frame "NUMPAD_9" {
          }
          frame "PAUSE" {
          }
          frame "PERIOD" {
          }
          frame "PRIOR (PG UP)" {
          }
          frame "RBRACKET" {
          }
          frame "RCONTROL" {
          }
          frame "RETURN" {
          }
          frame "R ALT" {
          }
          frame "RSHIFT" {
          }
          frame "RWIN" {
          }
          frame "SCROLL" {
          }
          frame "SEMICOLON" {
          }
          frame "SLASH" {
          }
          frame "SPACE" {
          }
          frame "SUBTRACT" {
          }
          frame "TAB" {
          }
          frame "DIVIDE" {
          }
          frame "DELETE" {
          }
          frame "DECIMAL" {
          }
          frame "COMMA" {
          }
          frame "CAPITAL" {
          }
          frame "BACKSLASH" {
          }
          frame "BACK" {
          }
          frame "ADD" {
          }
          frame "F15" {
          }
          frame "F14" {
          }
          frame "F13" {
          }
          frame "F12" {
          }
          frame "F11" {
          }
          frame "F10" {
          }
          frame "F9" {
          }
          frame "F8" {
          }
          frame "F7" {
          }
          frame "F6" {
          }
          frame "F5" {
          }
          frame "F4" {
          }
          frame "F3" {
          }
          frame "F2" {
          }
          frame "F1" {
          }
          frame "Z" {
          }
          frame "Y" {
          }
          frame "X" {
          }
          frame "W" {
          }
          frame "V" {
          }
          frame "U" {
          }
          frame "T" {
          }
          frame "S" {
          }
          frame "R" {
          }
          frame "Q" {
          }
          frame "P" {
          }
          frame "O" {
          }
          frame "N" {
          }
          frame "M" {
          }
          frame "L" {
          }
          frame "K" {
          }
          frame "J" {
          }
          frame "I" {
          }
          frame "H" {
          }
          frame "G" {
          }
          frame "F" {
          }
          frame "E" {
          }
          frame "D" {
          }
          frame "C" {
          }
          frame "B" {
          }
          frame "A" {
          }
          frame "9" {
          }
          frame "8" {
          }
          frame "7" {
          }
          frame "6" {
          }
          frame "5" {
          }
          frame "4" {
          }
          frame "3" {
          }
          frame "2" {
          }
          frame "1" {
          }
          frame "0" {
          }
        }
        n122 = property on="Previous File" class="Bool (strict)"(error in=w162, "Value"=w155) -> (error out=w161:errorcluster)  [unwired: 1 in, 1 out]
        n123 = Bundle(w139, w140, w125, w126, 0.0) -> (w127:cluster{dbl, dbl, dbl, dbl, dbl})  [unwired: 1 in]
        n124 = Divide(x=20.0, y=w151) -> (x/y=w149:dbl)
        n125 = Bundle("X"=w119, "Y"=w120) -> (w123:cluster{"X":sgl, "Y":sgl})  [unwired: 1 in]
        n126 = call "IMAQ Convert Rectangle to ROI (Polygon)"("Rectangle"=w127) -> ("ROI Descriptor"=w129:T14)  [unwired: 7 in, 2 out]
        n127 = property on="Save" class="Bool (strict)"(error in=w161, "Value"=w155) -> (error out=w160:errorcluster)  [unwired: 1 in, 1 out]
        n128 = property on="Export" class="Bool (strict)"("Value"=w155) -> ()  [unwired: 2 in, 2 out]
        n129 = property on="Image Out" class="ImageControl"("Image Center Position"=w123) -> ()  [unwired: 2 in, 2 out]
        n130 = property on="Image Preview" class="ImageControl"("ROI"=w129) -> ()  [unwired: 2 in, 2 out]
        n131 = property on="Save Next" class="Bool (strict)"(error in=w160, "Value"=w155) -> (error out=w159:errorcluster)  [unwired: 1 in, 1 out]
        n132 = property on="Discard" class="Bool (strict)"(error in=w159, "Value"=w155) -> (error out=w158:errorcluster)  [unwired: 1 in, 1 out]
        n133 = property on="Save Lines" class="Bool (strict)"(error in=w158, "Value"=w155) -> ()  [unwired: 1 in, 2 out]
        n134 = property on="Close" class="Bool (strict)"("Value"=w155) -> ()  [unwired: 2 in, 2 out]
        n135 = Bundle("Application Font", w149, w145, w145, w145, w145, w145, TRUE, w147) -> (w144:T15)  [unwired: 1 in]
        n136 = property on="Disable Flag" class="Bool (strict)"("Value"=w155) -> ()  [unwired: 2 in, 2 out]
        n137 = Bundle(w147, w144, w147, w147) -> (w101:T16)  [unwired: 1 in]
        n138 = Cluster To Array(cluster=w154) -> (array=w172:bool[])
        n139 = local read "Image Out"() -> (w100:T8)
        n140 = property on="Image Out" class="ImageControl"() -> ("ROI"=w103:T17)  [unwired: 2 in, 2 out]
        n141 = Unbundle By Name(w103) -> ("Contours"=w104:T18)
        n142 = call "IMAQ Clear Overlay"("Image"=w100) -> ("Image Out"=w117:T8)  [unwired: 9 in, 1 out]
        n143 = Initialize Array(0) -> (w106:i32[])  [unwired: 1 in]
        n144 = Array Size(array=w104) -> (size(s)=w105:i32)
        n145 = call "Next State.vi"("Buttons []"=w172, "States []"=w173) -> ("Save Next?"=→"Save Next?":bool, "Enum"=w165:T2)
        n146 = event shown="[1] \"New: Dielectric\", \"New: Width\", \"New: Length\", \"New: Temp\", \"New: Comments\": Value Change" {
          selector: _ -> [_ _ _ _ _ _ _ _ _ _ _ _ _ _ _]
          dyn-events: _ -> [_ _ _ _ _ _ _ _ _ _ _ _ _ _ _]
          timeout: 5 -> [_ _ _ _ _ _ _ _ _ _ _ _ _ _ _]
          tunnel: w165 -> [w428 _ _ _ _ _ _ _ _ _ _ _ _ _ _]
          tunnel: [w428 MegaAwesome_States."Re-Calculated Values" MegaAwesome_States."Calculated Values" MegaAwesome_States."Re-Calculated Values" MegaAwesome_States."Re-Calculated Values" MegaAwesome_States."Re-Calculated Values" MegaAwesome_States."Re-Calculated Values" MegaAwesome_States."Read Data" MegaAwesome_States."Read Data" MegaAwesome_States."No Event" MegaAwesome_States."No Event" MegaAwesome_States."No Event" MegaAwesome_States."No Event" MegaAwesome_States."No Event" MegaAwesome_States."No Event"] -> w164
          tunnel: w89 -> [w427 w429 w431 w433 w458 w486 w510 _ w538 w540 w553 w555 w559 w563 w567]
          tunnel: [w427 w429 w431 w433 w458 w486 w510 w529 w538 w540 w553 w555 w559 w563 w567] -> w157
          tunnel: w156 -> [_ _ _ _ _ _ _ w528 _ _ _ _ _ _ _]
          tunnel: w154 -> [_ _ _ _ _ _ _ _ _ _ _ _ _ _ _]
          event Timeout {
            n147 = event-data() -> ()  [unwired: 1 in, 2 out]
          }
          event "New: Dielectric", "New: Width", "New: Length", "New: Temp", "New: Comments": Value Change {
            n148 = event-data() -> ()  [unwired: 1 in, 5 out]
          }
          event "Num Pts Log", "Transport Style Controls", "Num Pts": Value Change {
            n149 = event-data() -> ()  [unwired: 1 in, 5 out]
          }
          event "Sat-Trans Slider": Value Change {
            n150 = event-data() -> ()  [unwired: 1 in, 5 out]
            n151 = local read "Sqrt-Sat"() -> (w457:cluster{dbl[], dbl[]}[])
            n152 = Decimate 1D Array(w457) -> (w441:cluster{dbl[], dbl[]}[], w442:cluster{dbl[], dbl[]}[])
            n153 = local read "Slider Min"() -> (w438:dbl)
            n154 = local read "Sat-Trans Slider"() -> (w436:dbl)
            n155 = Array To Cluster(array=w441) -> (cluster=w456:T19)
            n156 = local read "New: Dielectric"() -> (w451:dbl)
            n157 = local read "Num Pts"() -> (w434:dbl)
            n158 = local read "New: Width"() -> (w453:dbl)
            n159 = local read "New: Length"() -> (w452:dbl)
            n160 = Unbundle(w456) -> ("[0]"=w455:cluster{dbl[], dbl[]})  [unwired: 8 out]
            n161 = Absolute Value(x=w438) -> (abs(x)=w437:dbl)
            n162 = Unbundle(w455) -> (w439:dbl[], w454:dbl[])
            n163 = Add(x=w436, y=w437) -> (x+y=w435:dbl)
            n164 = Array Subset(array=w439, index=w435, length=w434) -> (w449:dbl[])
            n165 = local write "Sat Vg Array-Used"(w449) -> ()
            n166 = Array Subset(array=w454, index=w435, length=w434) -> (w450:dbl[])
            n167 = call "Mobility-Vt-Used Pts_Saturation.vi"("Width"=w453, "Length"=w452, "Dielectric (d)"=w451, "Sat Id Used"=w450, "Vg Used"=w449) -> ("Vt"=w445:dbl, "Mobility"=w446:dbl)  [unwired: 4 in, 1 out]
            n168 = local write "Index-Sat"(w435) -> ()
            n169 = local write "Sat Id-Used"(w450) -> ()
            n170 = Bundle(w449, w450) -> (w443:cluster{dbl[], dbl[]})  [unwired: 1 in]
            n171 = local read "Re-Calculated Values Cluster"() -> (w448:T9)
            n172 = Bundle By Name(cluster=w448, "Mobility-Sat"=w446, "Vt-Sat"=w445) -> (w447:T9)
            n173 = local write "Re-Calculated Values Cluster"(w447) -> ()
            n174 = Build Array (concatenate)(w441, w442, w443) -> (w440:cluster{dbl[], dbl[]}[])
            n175 = local write "Sqrt-Sat"(w440) -> ()
          }
          event "Lin-Trans Slider": Value Change {
            n176 = event-data() -> ()  [unwired: 1 in, 5 out]
            n177 = local read "Sqrt-Lin"() -> (w482:cluster{dbl[], dbl[]}[])
            n178 = Decimate 1D Array(w482) -> (w467:cluster{dbl[], dbl[]}[], w468:cluster{dbl[], dbl[]}[])
            n179 = local read "Slider Min"() -> (w464:dbl)
            n180 = Array To Cluster(array=w467) -> (cluster=w481:T19)
            n181 = local read "Lin-Trans Slider"() -> (w462:dbl)
            n182 = local read "New: Dielectric"() -> (w475:dbl)
            n183 = local read "Num Pts"() -> (w478:dbl)
            n184 = local read "New: Width"() -> (w477:dbl)
            n185 = local read "New: Length"() -> (w476:dbl)
            n186 = local read "Lin Vd"() -> (w459:dbl)
            n187 = Unbundle(w481) -> ("[0]"=w480:cluster{dbl[], dbl[]})  [unwired: 8 out]
            n188 = Absolute Value(x=w464) -> (abs(x)=w463:dbl)
            n189 = Unbundle(w480) -> (w465:dbl[], w479:dbl[])
            n190 = Add(x=w462, y=w463) -> (x+y=w461:dbl)
            n191 = Array Subset(array=w465, index=w461, length=w478) -> (w473:dbl[])
            n192 = local write "Lin-Vg Array-Used"(w473) -> ()
            n193 = Array Subset(array=w479, index=w461, length=w478) -> (w474:dbl[])
            n194 = call "Mobility-Vt-Used Pts_Linear.vi"("Width"=w477, "Length"=w476, "Vd"=w459, "Dielectric (d)"=w475, "Id Used"=w474, "Vg Used"=w473) -> ("Mobility"=w470:dbl)  [unwired: 3 in, 2 out]
            n195 = local write "Index-Lin"(w461) -> ()
            n196 = local write "Lin Id-Used"(w474) -> ()
            n197 = Bundle(w473, w474) -> (w469:cluster{dbl[], dbl[]})  [unwired: 1 in]
            n198 = local read "Re-Calculated Values Cluster"() -> (w472:T9)
            n199 = Bundle By Name(cluster=w472, "Moblitity-Lin"=w470) -> (w471:T9)
            n200 = local write "Re-Calculated Values Cluster"(w471) -> ()
            n201 = Build Array (concatenate)(w467, w468, w469) -> (w466:cluster{dbl[], dbl[]}[])
            n202 = local write "Sqrt-Lin"(w466) -> ()
          }
          event "Sat-Log Slider": Value Change {
            n203 = event-data() -> ()  [unwired: 1 in, 5 out]
            n204 = local read "Sat-Log"() -> (w489:cluster{dbl[], dbl[]}[])
            n205 = Decimate 1D Array(w489) -> (w496:cluster{dbl[], dbl[]}[], w497:cluster{dbl[], dbl[]}[])
            n206 = local read "Slider Min"() -> (w493:dbl)
            n207 = Array To Cluster(array=w496) -> (cluster=w506:T19)
            n208 = property on="Sat-Log" class="XYGraph (strict)"("Active Plot"=2, "Plot.Fill/Pt. Color"=u32 6618880, "Plot.Point Style"=11) -> ()  [unwired: 2 in, 2 out]
            n209 = local read "Num Pts Log"() -> (w503:dbl)
            n210 = local read "Sat-Log Slider"() -> (w491:dbl)
            n211 = Unbundle(w506) -> ("[0]"=w505:cluster{dbl[], dbl[]})  [unwired: 8 out]
            n212 = Absolute Value(x=w493) -> (abs(x)=w492:dbl)
            n213 = Unbundle(w505) -> (w494:dbl[], w504:dbl[])
            n214 = Add(x=w491, y=w492) -> (x+y=w488:dbl)
            n215 = Array Subset(array=w494, index=w488, length=w503) -> (w501:dbl[])
            n216 = Array Subset(array=w504, index=w488, length=w503) -> (w502:dbl[])
            n217 = local write "Vg Array-Log-Used"(w501) -> ()
            n218 = local write "IndexLog-Sat"(w488) -> ()
            n219 = Bundle(w501, w502) -> (w487:cluster{dbl[], dbl[]})  [unwired: 1 in]
            n220 = call "STS-Used.vi"("Id Used"=w502, "Vg-Used"=w501) -> ("STS"=w498:dbl)  [unwired: 9 in]
            n221 = local write "Sat Id-Log-Used"(w502) -> ()
            n222 = local read "Re-Calculated Values Cluster"() -> (w500:T9)
            n223 = Bundle By Name(cluster=w500, "STS"=w498) -> (w499:T9)
            n224 = local write "Re-Calculated Values Cluster"(w499) -> ()
            n225 = Build Array (concatenate)(w496, w497, w487) -> (w495:cluster{dbl[], dbl[]}[])
            n226 = local write "Sat-Log"(w495) -> ()
          }
          event "Lin-Log Slider": Value Change {
            n227 = event-data() -> ()  [unwired: 1 in, 5 out]
            n228 = local read "Lin-Log"() -> (w514:cluster{dbl[], dbl[]}[])
            n229 = Decimate 1D Array(w514) -> (w520:cluster{dbl[], dbl[]}[], w521:cluster{dbl[], dbl[]}[])
            n230 = local read "Slider Min"() -> (w517:dbl)
            n231 = Array To Cluster(array=w520) -> (cluster=w527:T19)
            n232 = local read "Num Pts Log"() -> (w524:dbl)
            n233 = property on="Lin-Log" class="XYGraph (strict)"("Active Plot"=2, "Plot.Fill/Pt. Color"=u32 6618880, "Plot.Point Style"=11) -> ()  [unwired: 2 in, 2 out]
            n234 = local read "Lin-Log Slider"() -> (w515:dbl)
            n235 = Unbundle(w527) -> ("[0]"=w526:cluster{dbl[], dbl[]})  [unwired: 8 out]
            n236 = Absolute Value(x=w517) -> (abs(x)=w516:dbl)
            n237 = Unbundle(w526) -> (w518:dbl[], w525:dbl[])
            n238 = Add(x=w515, y=w516) -> (x+y=w513:dbl)
            n239 = Array Subset(array=w518, index=w513, length=w524) -> (w522:dbl[])
            n240 = local write "Lin-Vg Array-Log Used"(w522) -> ()
            n241 = Array Subset(array=w525, index=w513, length=w524) -> (w523:dbl[])
            n242 = local write "IndexLog-Sat"(w513) -> ()
            n243 = Bundle(w522, w523) -> (w512:cluster{dbl[], dbl[]})  [unwired: 1 in]
            n244 = local write "Lin Id-Log Used"(w523) -> ()
            n245 = Build Array (concatenate)(w520, w521, w512) -> (w519:cluster{dbl[], dbl[]}[])
            n246 = local write "Lin-Log"(w519) -> ()
          }
          event "Index Array": Value Change {
            n247 = event-data() -> ()  [unwired: 1 in, 5 out]
            n248 = Strip Path(path=w528) -> (stripped path=w534:path)  [unwired: 1 out]
            n249 = local write "Transfer Folder"(w534) -> ()
            n250 = List Folder(path=w534) -> (filenames=w530:string[])  [unwired: 3 in, 3 out]
            n251 = local read "Index Array"() -> (w529:i32)
            n252 = Path To String(path=w534) -> (string=w535:string)
            n253 = Index Array(array=w530, index=w529) -> (element=w536:string)
            n254 = Concatenate Strings(w535, "\\", w536) -> (w532:string)
            n255 = String To Path(string=w532) -> (path=w531:path)
            n256 = local write "Transfer File"(w531) -> ()
          }
          event "Transfer File": Value Change {
            n257 = event-data() -> ()  [unwired: 1 in, 5 out]
          }
          event "Remove Button": Mouse Down {
            w542 = 0
            n258 = event-data() -> ()  [unwired: 1 in, 5 out]
            n259 = property on="Image Out" class="ImageControl"() -> ("ROI"=w552:T17)  [unwired: 2 in, 2 out]
            n260 = Unbundle(w552) -> ("Global Rectangle"=w543:i32[], "Contours"=w545:T18)
            n261 = Reverse 1D Array(array=w543) -> (reversed array=w544:i32[])
            n262 = Reverse 1D Array(array=w545) -> (reversed array=w546:T18)
            n263 = Delete From Array(array=w544, index=w542) -> (array with subset deleted=w547:i32[])  [unwired: 1 in, 1 out]
            n264 = Delete From Array(array=w546, index=w542) -> (array with subset deleted=w548:T18)  [unwired: 1 in, 1 out]
            n265 = Reverse 1D Array(array=w547) -> (reversed array=w549:i32[])
            n266 = Reverse 1D Array(array=w548) -> (reversed array=w550:T18)
            n267 = Bundle(w549, w550) -> (w551:T20)  [unwired: 1 in]
            n268 = property on="Image Out" class="ImageControl"("ROI"=w551) -> ()  [unwired: 2 in, 2 out]
          }
          event "Undo Button": Mouse Down {
            n269 = event-data() -> ()  [unwired: 1 in, 5 out]
            n270 = invoke on="Image Out" class="ImageControl" method="Clear ROI"() -> ()  [unwired: 3 in, 3 out]
          }
          event "Image Folder": Value Change {
            n271 = event-data() -> ()  [unwired: 1 in, 5 out]
            n272 = local read "Image File"() -> (w557:path)
            n273 = call "Vision Acquisition"("Image Path"=w557) -> ("Image Out"=w558:T8)  [unwired: 25 in, 1 out]
            n274 = local write "Image Preview"(w558) -> ()
            n275 = local write "Image Out"(w558) -> ()
          }
          event "Zoom": Value Change {
            n276 = event-data() -> ()  [unwired: 1 in, 5 out]
            n277 = local read "Zoom"() -> (w562:i32)
            n278 = Bundle("Zoom"=w562, "Zoom"=w562) -> (w561:cluster{"Zoom":i32, "Zoom":i32})  [unwired: 1 in]
            n279 = property on="Image Out" class="ImageControl"("ZoomInteger"=w561) -> ()  [unwired: 2 in, 2 out]
          }
          event "Image Out": Mouse Enter {
            n280 = event-data() -> ()  [unwired: 1 in, 3 out]
            n281 = call "Simulate_Keyboard.vi"("Action"=0, "Virtual Key"=162) -> ()  [unwired: 7 in, 1 out]
          }
          event "Image Out": Mouse Leave {
            n282 = event-data() -> ()  [unwired: 1 in, 3 out]
            n283 = flat-sequence {
              frame #0 {
                n284 = Wait (ms)(milliseconds to wait=10) -> ()  [unwired: 1 out]
              }
              frame #1 {
                n285 = call "Simulate_Keyboard.vi"("Action"=2, "Virtual Key"=162) -> ()  [unwired: 7 in, 1 out]
              }
            }
          }
        }
        n286 = Build Array(0.505025, 0.252522, 0.127742, 0.050345, 0.031129) -> (w113:dbl[])
        n287 = Array Subset(array=w113, index="Magnification", length=1) -> (w115:dbl[])
        n288 = To Double Precision Float(number=w115) -> (double precision float=w116:dbl[])
        n289 = for {
          N: w105 -> [_]
          shift-right: [w199] -> _
          shift-left: w104 -> [w199]
          shift-right: [w175] -> w91
          shift-left: w106 -> [w197]
          tunnel: w116 -> [w196]
          shift-right: [w193] -> _
          shift-left: w117 -> [w195]
          tunnel: w101 -> [w189]
          i -> [w192]
          n290 = Index Array(array=w199, index=w192) -> (element=w208:T21)
          n291 = Unbundle(w208) -> ("Points"=w207:i32[])  [unwired: 2 out]
          n292 = Array To Cluster(array=w207) -> (cluster=w206:T22)
          n293 = Unbundle(w206) -> ("Points[0]"=w188:i32, "Points[1]"=w185:i32, "Points[2]"=w198:i32, "Points[3]"=w204:i32)  [unwired: 5 out]
          n294 = Add(x=w188, y=10) -> (x+y=w186:i32)
          n295 = Subtract(x=w185, y=w204) -> (x-y=w203:i32)
          n296 = Subtract(x=w188, y=w198) -> (x-y=w205:i32)
          n297 = Square(x=w203) -> (x^2=w201:i32)
          n298 = Square(x=w205) -> (x^2=w202:i32)
          n299 = Add(x=w202, y=w201) -> (x+y=w200:i32)
          n300 = Square Root(x=w200) -> (sqrt(x)=w179:dbl)
          n301 = Multiply(x=w179, y=0.5) -> (x*y=w182:dbl)
          n302 = Multiply(x=w179, y=w196) -> (x*y=w178:dbl[])
          n303 = Index Array(array=w178) -> (element=w191:dbl)  [unwired: 1 in]
          n304 = Number To Fractional String(number=w191, precision (6)=0) -> (F-format string=w190:string)  [unwired: 2 in]
          n305 = Build Array (concatenate)(w197, w178) -> (w176:dbl[])
          n306 = Add(x=w182, y=w185) -> (x+y=w184:dbl)
          n307 = Bundle(w186, w184) -> (w194:cluster{i32, dbl})  [unwired: 1 in]
          n308 = call "IMAQ Overlay Text"("BG Color (Transparent)"=u32 0, "Text Color (black)"=u32 16448250, "Font, Size & Style"=w189, "String"=w190, "Origin"=w194, "Image"=w195) -> ("Image Out"=w193:T8)  [unwired: 4 in, 1 out]
          n309 = To Long Integer(number=w176) -> (32bit integer=w175:i32[])
        }
        "Distances" <- w91
        n310 = Add Array Elements(numeric array=w91) -> (sum=w102:i32)
        n311 = local write "Total Width"(w102) -> ()
      }
      frame "Read Data" {
        n312 = call "IMAQ Dispose"("All Images? (No)"=TRUE) -> ()  [unwired: 5 in, 1 out]
        n313 = case shown="True" "Disable Flag" {
          tunnel: w617 -> [_ w642]
          tunnel: [w638 w639] -> w616
          tunnel: w614 -> [w638 _]
          frame False {
          }
          frame True {
            n314 = local read "Transfer Folder"() -> (w641:path)
            n315 = List Folder(path=w641) -> (filenames=w643:string[])  [unwired: 3 in, 3 out]
            n316 = Index Array(array=w643, index=w642) -> (element=w640:string)
            n317 = Build Path(base path=w641, name or relative path=w640) -> (appended path=w639:path)
            n318 = local write "Transfer File"(w639) -> ()
          }
        }
        n319 = call "Recorded Values.vi"("Path"=w616) -> ("Recorded Char"=→"Recorded Values Cluster":T9, "Recorded Prop"=w629:T1, "Fabrication Prop"=w627:T4)  [unwired: 8 in]
        n320 = Strip Path(path=w616) -> (stripped path=w626:path, name=w625:string)
        n321 = local write "Fabrication Prop"(w627) -> ()
        n322 = local write "Recorded Prop"(w629) -> ()
        n323 = Unbundle By Name(w629) -> ("Date Recorded"=→"Date Recorded":string, "Index"=w628:string, "Length"=w622:dbl, "Width"=w621:dbl)  [unwired: 1 out]
        n324 = Unbundle By Name(w629) -> ("Sample Temp"=w631:dbl)
        n325 = Unbundle By Name(w627) -> ("Dielectric (nm)"=w623:dbl, "Comments"=w624:string, "Date Created"=→"Date Created":string)
        n326 = List Folder(path=w626) -> (filenames=w620:string[])  [unwired: 3 in, 3 out]
        n327 = local write "Rec: Dielectric (d)"(w623) -> ()
        n328 = local write "Index"(w628) -> ()
        n329 = local write "Rec: Length"(w622) -> ()
        n330 = local write "Rec: Width"(w621) -> ()
        n331 = Equal To 0?(x=w631) -> (x = 0?=w634:bool)
        n332 = Number To Decimal String(number=w631) -> (decimal integer string=w635:string)  [unwired: 1 in]
        n333 = local write "Comments:"(w624) -> ()
        n334 = Search 1D Array(1D array=w620, element=w625) -> (index of element=w619:i32)  [unwired: 1 in]
        n335 = Equal?(x="", y=w635) -> (x = y?=w633:bool)
        n336 = Index Array(array=w620, index=w619) -> (element=→"Data Name:":string)
        n337 = local write "New: Width"(w621) -> ()
        n338 = local write "New: Length"(w622) -> ()
        n339 = local write "Index Array"(w619) -> ()
        n340 = Or(x=w634, y=w633) -> (x .or. y?=w632:bool)
        n341 = local write "New: Dielectric"(w623) -> ()
        n342 = case shown="True" w632 {
          tunnel: [w644 w645] -> w613
          tunnel: w631 -> [w644 _]
          frame False {
          }
          frame True {
            n343 = local read "Room Temp"() -> (w645:dbl)
          }
        }
        n344 = local write "New: Temp"(w613) -> ()
        n345 = Bundle By Name(cluster=w629, "Sample Temp"=w613) -> (w630:T1)
        n346 = local write "Rec: Temp"(w613) -> ()
        n347 = local write "Recorded Prop"(w630) -> ()
      }
      frame "Calculated Values" {
        n348 = local read "Image Center X"() -> (w647:i32)
        n349 = call "Image from TRF Display.vi"("Image Center X"=w647, "No Image File"=w692, "Image Folder"=w693, "Transfer File"=w662) -> ("Image Preview"=w654:T8, "Image Out"=w655:T8, "Image File"=w656:path, "Image Name"=→"Image Name":string, "ROI File"=w651:path)  [unwired: 3 in]
        n350 = invoke on="Image Out" class="ImageControl" method="Clear ROI"() -> ()  [unwired: 3 in, 3 out]
        n351 = local write "Image File"(w656) -> ()
        n352 = local write "Image Out"(w655) -> ()
        n353 = local write "Image Preview"(w654) -> ()
        n354 = call <vilib>:"Check if File or Folder Exists.vi"("path"=w651) -> ("file or folder exists?"=w652:bool, "dup path"=w653:path)  [unwired: 8 in, 1 out]
        n355 = case shown="True" w652 {
          tunnel: w653 -> [_ w713]
          frame False {
          }
          frame True {
            n356 = Read from Text File(file (use dialog)=w713) -> (text=w717:string)  [unwired: 3 in, 3 out]
            n357 = property on="Image Out" class="ImageControl"() -> ("ROI"=w714:T17)  [unwired: 2 in, 2 out]
            n358 = Unflatten From String(type=w714, binary string=w717) -> (value=w715:T17, error out=w716:errorcluster)  [unwired: 3 in, 1 out]
            n359 = property on="Image Out" class="ImageControl"(error in=w716, "ROI"=w715) -> ()  [unwired: 1 in, 2 out]
          }
        }
        n360 = call "TRF to TSP Plot_09_21_12a_JW.vi"("Transport Graph Properties"="Transport Style Controls", "No Transport File"=w657, "Transport Folder"=w658, "Transfer File"=w662) -> ("Transport"=w663:cluster{ext[], ext[]}[], "Transport File"=→"Transport\nFile":path, "Transport Name"=→"Transport Name:":string)  [unwired: 5 in]
        "Transport" <- w663
        n361 = Array Size(array=w663) -> (size(s)=w661:i32)
        n362 = local read "Image Center X"() -> (w648:i32)
        n363 = for {
          N: w661 -> [_]
          tunnel: "Transport Style Controls" -> [w721]
          i -> [w720]
          n364 = Unbundle By Name(w721) -> ("Transport Line Size"=w718:u16, "Transport Line Color"=w719:u32)
          n365 = property on="Transport" class="XYGraph (strict)"("Active Plot"=w720, "Plot.Plot Color"=w719, "Plot.Line Width"=w718) -> ()  [unwired: 2 in, 2 out]
        }
        n366 = local read "Recorded Prop"() -> (w695:T1)
        n367 = local read "Fabrication Prop"() -> (w702:T4)
        n368 = Bundle("Image Center X"=w648, 0) -> (w650:cluster{"Image Center X":i32, i32})  [unwired: 1 in]
        n369 = property on="Image Out" class="ImageControl"("Image Center Position"=w650) -> ()  [unwired: 2 in, 2 out]
        n370 = local read "Calculated Values Cluster"() -> (w712:T9)
        n371 = call "Mobility-Vt Calculator-File.vi"("NumPts"=w697, "Path"=w662) -> ("Used Points"=w690:T23, "Graph Cluster"=w680:T24, "Lin Vd"=w665:dbl, "Output"=w710:T25)  [unwired: 6 in]
        n372 = call "STS Calculator-File.vi"("NumPts"=w696, "Path"=w662) -> ("Used Points"=w685:T26, "XY Graph-Sat"=w669:cluster{dbl[], dbl[]}[], "XY Graph-Lin"=w666:cluster{dbl[], dbl[]}[], "Ouput"=w705:cluster{"STS-Sat":dbl, "STS-Lin":dbl})  [unwired: 6 in]
        n373 = Unbundle By Name(w702) -> ("Dielectric (nm)"=w700:dbl)
        n374 = Unbundle By Name(w695) -> ("Sample Temp"=w694:dbl)
        n375 = Unbundle By Name(w710) -> ("Mobility-Sat"=w709:dbl, "Vt-Sat"=w701:dbl, "Mobility-Lin"=w708:dbl, "Off I-Sat"=w707:dbl, "On/Off I-Sat"=w706:dbl)  [unwired: 1 out]
        n376 = local write "Lin Vd"(w665) -> ()
        n377 = Unbundle By Name(w705) -> ("STS-Sat"=w699:dbl)  [unwired: 1 out]
        n378 = local write "Sat-Log"(w669) -> ()
        n379 = local write "Lin-Log"(w666) -> ()
        n380 = call "Trap Density_VT.vi"("VT"=w701, "Dielectric"=w700) -> ("Trap Density-VT"=w704:dbl)
        n381 = call "Trap Density_STS.vi"("Temp (T) [K]"=w694, "S.T.S. (S)"=w699, "Dielectric"=w700) -> ("Trap Density (N)"=w703:dbl)  [unwired: 8 in]
        n382 = Bundle By Name(cluster=w712, "Mobility-Sat"=w709, "Moblitity-Lin"=w708, "On/Off"=w706, "Off Current"=w707, "Vt-Sat"=w701, "STS"=w699, "Trap Density-VT"=w704, "Trap Density-STS"=w703) -> (w711:T9)
        n383 = Unbundle By Name(w685) -> ("Sat Vg Used"=w684:dbl[], "Sat Log(Id) Used"=w683:dbl[], "Lin Vg Used"=w682:dbl[], "Lin Log(Id) Used"=w681:dbl[], "STS Index-Sat"=w667:dbl, "STS Index-Lin"=w668:dbl)
        n384 = Unbundle By Name(w690) -> ("Sat Vg Used"=w689:dbl[], "Sat Sqrt(Id) Used"=w688:dbl[], "Lin Vg Used"=w687:dbl[], "Lin Sqrt(Id) Used"=w686:dbl[], "Index-Lin"=w676:dbl, "Index-Sat"=w675:dbl)
        n385 = local write "Vg Array-Log-Used"(w684) -> ()
        n386 = local write "Sat Id-Log-Used"(w683) -> ()
        n387 = local write "Lin-Vg Array-Log Used"(w682) -> ()
        n388 = local write "Lin Id-Log Used"(w681) -> ()
        n389 = local write "IndexLog-Sat"(w667) -> ()
        n390 = local write "Index-Lin"(w668) -> ()
        n391 = local write "Calculated Values Cluster"(w711) -> ()
        n392 = local write "Sat Vg Array-Used"(w689) -> ()
        n393 = local write "Sat Id-Used"(w688) -> ()
        n394 = local write "Lin-Vg Array-Used"(w687) -> ()
        n395 = local write "Lin Id-Used"(w686) -> ()
        n396 = local write "Index-Sat"(w675) -> ()
        n397 = local write "Index-Lin"(w676) -> ()
        n398 = local write "Lin-Log Slider"(w668) -> ()
        n399 = local write "Sat-Log Slider"(w667) -> ()
        n400 = local write "Sat-Trans Slider"(w675) -> ()
        n401 = local write "Lin-Trans Slider"(w676) -> ()
        n402 = Unbundle By Name(w680) -> ("Raw Sat"=w674:cluster{dbl[], dbl[]}[], "Sqrt Sat"=w677:cluster{dbl[], dbl[]}[], "Raw Lin"=w679:cluster{dbl[], dbl[]}[], "Sqrt Lin"=w678:cluster{dbl[], dbl[]}[])
        n403 = Index Array(array=w674) -> (element=w673:cluster{dbl[], dbl[]})  [unwired: 1 in]
        n404 = Unbundle(w673) -> (w672:dbl[])  [unwired: 1 out]
        n405 = Array Max & Min(array=w672) -> (max value=w671:dbl, min value=w670:dbl)  [unwired: 2 out]
        n406 = property on="Sat-Trans Slider" class="Slide (strict)"("Scale.Maximum"=w671, "Scale.Minimum"=w670) -> ()  [unwired: 2 in, 2 out]
        n407 = property on="Lin-Trans Slider" class="Slide (strict)"("Scale.Maximum"=w671, "Scale.Minimum"=w670) -> ()  [unwired: 2 in, 2 out]
        n408 = property on="Sat-Log Slider" class="Slide (strict)"("Scale.Maximum"=w671, "Scale.Minimum"=w670) -> ()  [unwired: 2 in, 2 out]
        n409 = property on="Lin-Log Slider" class="Slide (strict)"("Scale.Maximum"=w671, "Scale.Minimum"=w670) -> ()  [unwired: 2 in, 2 out]
        n410 = local write "Slider Max"(w671) -> ()
        n411 = local write "Slider Min"(w670) -> ()
        n412 = local write "Raw- Sat"(w674) -> ()
        n413 = local write "Raw- Lin"(w679) -> ()
        n414 = local write "Sqrt-Sat"(w677) -> ()
        n415 = local write "Sqrt-Lin"(w678) -> ()
      }
      frame "Re-Calculated Values" {
        n416 = local read "Vg Array-Log-Used"() -> (w730:dbl[])
        n417 = local read "Sat Vg Array-Used"() -> (w738:dbl[])
        n418 = local read "Lin-Vg Array-Used"() -> (w744:dbl[])
        n419 = local read "Sat Id-Log-Used"() -> (w729:dbl[])
        n420 = local read "New: Dielectric"() -> (w742:dbl)
        n421 = local read "New: Dielectric"() -> (w727:dbl)
        n422 = local read "New: Length"() -> (w741:dbl)
        n423 = local read "New: Length"() -> (w737:dbl)
        n424 = local read "New: Width"() -> (w740:dbl)
        n425 = local read "New: Width"() -> (w736:dbl)
        n426 = local read "Lin Id-Used"() -> (w743:dbl[])
        n427 = local read "Sat Id-Used"() -> (w735:dbl[])
        n428 = local read "Re-Calculated Values Cluster"() -> (w746:T9)
        n429 = local read "New: Dielectric"() -> (w726:dbl)
        n430 = local read "New: Temp"() -> (w725:dbl)
        n431 = local read "Lin Vd"() -> (w722:dbl)
        n432 = call "Mobility-Vt-Used Pts_Saturation.vi"("Width"=w736, "Length"=w737, "Dielectric (d)"=w727, "Sat Id Used"=w735, "Vg Used"=w738) -> ("Vt"=w733:dbl, "Mobility"=w734:dbl)  [unwired: 4 in, 1 out]
        n433 = call "STS-Used.vi"("Id Used"=w729, "Vg-Used"=w730) -> ("STS"=w728:dbl)  [unwired: 9 in]
        n434 = call "Mobility-Vt-Used Pts_Linear.vi"("Width"=w740, "Length"=w741, "Vd"=w722, "Dielectric (d)"=w742, "Id Used"=w743, "Vg Used"=w744) -> ("Mobility"=w739:dbl)  [unwired: 3 in, 2 out]
        n435 = call "Trap Density_VT.vi"("VT"=w733, "Dielectric"=w727) -> ("Trap Density-VT"=w732:dbl)
        n436 = call "Trap Density_STS.vi"("Temp (T) [K]"=w725, "S.T.S. (S)"=w728, "Dielectric"=w726) -> ("Trap Density (N)"=w724:dbl)  [unwired: 8 in]
        n437 = Bundle By Name(cluster=w746, "Mobility-Sat"=w734, "Moblitity-Lin"=w739, "Vt-Sat"=w733, "STS"=w728, "Trap Density-VT"=w732, "Trap Density-STS"=w724) -> (w745:T9)
        n438 = local write "Re-Calculated Values Cluster"(w745) -> ()
      }
      frame "Next File" {
        n439 = call "IMAQ Dispose"("All Images? (No)"=TRUE) -> ()  [unwired: 5 in, 1 out]
        n440 = Strip Path(path=w763) -> (stripped path=w754:path, name=w761:string)
        n441 = local write "Transfer Folder"(w754) -> ()
        n442 = List Folder(path=w754) -> (filenames=w748:string[])  [unwired: 3 in, 3 out]
        n443 = Array Size(array=w748) -> (size(s)=w760:i32)
        n444 = Search 1D Array(1D array=w748, element=w761) -> (index of element=w758:i32)  [unwired: 1 in]
        n445 = Decrement(x=w760) -> (x-1=w759:i32)
        n446 = Equal?(x=w759, y=w758) -> (x = y?=w757:bool)
        n447 = case shown="True" w757 {
          tunnel: w750 -> [w765 _]
          tunnel: [w764 0] -> w749
          frame False {
            n448 = Increment(x=w765) -> (x+1=w764:i32)
          }
          frame True {
          }
        }
        n449 = Path To String(path=w754) -> (string=w755:string)
        n450 = Index Array(array=w748, index=w749) -> (element=w756:string)
        n451 = Concatenate Strings(w755, "\\", w756) -> (w752:string)
        n452 = String To Path(string=w752) -> (path=w751:path)
        n453 = local write "Transfer File"(w751) -> ()
      }
      frame "Previous File" {
        n454 = call "IMAQ Dispose"("All Images? (No)"=TRUE) -> ()  [unwired: 5 in, 1 out]
        n455 = Strip Path(path=w774) -> (stripped path=w771:path, name=w782:string)
        n456 = local write "Transfer Folder"(w771) -> ()
        n457 = List Folder(path=w771) -> (filenames=w775:string[])  [unwired: 3 in, 3 out]
        n458 = Array Size(array=w775) -> (size(s)=w769:i32)
        n459 = Search 1D Array(1D array=w775, element=w782) -> (index of element=w781:i32)  [unwired: 1 in]
        n460 = Decrement(x=w769) -> (x-1=w768:i32)
        n461 = Equal To 0?(x=w781) -> (x = 0?=w780:bool)
        n462 = case shown="True" w780 {
          tunnel: w773 -> [w785 _]
          tunnel: [w784 w786] -> w772
          tunnel: w768 -> [_ w786]
          frame False {
            n463 = Decrement(x=w785) -> (x-1=w784:i32)
          }
          frame True {
          }
        }
        n464 = Path To String(path=w771) -> (string=w770:string)
        n465 = Index Array(array=w775, index=w772) -> (element=w779:string)
        n466 = Concatenate Strings(w770, "\\", w779) -> (w777:string)
        n467 = String To Path(string=w777) -> (path=w776:path)
        n468 = local write "Transfer File"(w776) -> ()
      }
      frame "Discard File" {
        n469 = Strip Path(path=w801) -> (stripped path=w796:path, name=w795:string)
        n470 = property on="Disable Flag" class="Bool (strict)"("Value"=TRUE) -> ()  [unwired: 2 in, 2 out]
        n471 = List Folder(path=w796) -> (filenames=w794:string[])  [unwired: 3 in, 3 out]
        n472 = Search 1D Array(1D array=w794, element=w795) -> (index of element=w798:i32)  [unwired: 1 in]
        n473 = call "IMAQ Dispose"("All Images? (No)"=TRUE) -> ()  [unwired: 5 in, 1 out]
        n474 = Strip Path(path=w801) -> (stripped path=w793:path, name=w792:string)
        n475 = String Subset(string=w792, offset (0)=0, length (rest)=1) -> (substring=w789:string)
        n476 = Equal?(x=w789, y="X") -> (x = y?=w787:bool)
        n477 = case shown="False" w787 {
          tunnel: w793 -> [w809 _]
          tunnel: w801 -> [w805 _]
          tunnel: w792 -> [w804 _]
          tunnel: w798 -> [w803 w813]
          tunnel: [w803 w812] -> w797
          frame False {
            n478 = Path To String(path=w809) -> (string=w808:string)
            n479 = Concatenate Strings(w808, "\\", "X_", w804) -> (w807:string)
            n480 = String To Path(string=w807) -> (path=w806:path)
            n481 = Move(source path=w805, 10:w806) -> ()  [unwired: 3 in, 3 out]
          }
          frame True {
            n482 = Increment(x=w813) -> (x+1=w812:i32)
          }
        }
      }
      frame "Save" {
        n483 = stacked-sequence {
          seq-local: [w828 _] -> [_ w1325]
          seq-local: [w827 _] -> [_ w1323]
          tunnel: w820 -> [w829 w1326]
          frame #0 {
            # "Saves each Re-calculated parameter in sequence"
            n484 = stacked-sequence {
              tunnel: [_ _ _ _ _ _ _ _ _ _ _ _ _ w1293] -> w827
              tunnel: w829 -> [w849 _ _ _ _ _ _ _ _ _ _ _ _ _]
              frame #0 {
                n485 = call-poly <vilib>:"Read From Spreadsheet File.vi"("file path (dialog if empty)"=w849) -> ("all rows"=w848:string[][])  [unwired: 6 in, 4 out]
                n486 = Array Size(array=w848) -> (size(s)=w853:i32[])
                n487 = Array Subset(array=w848, index (row)=0, index (col)=0, length (col)=3) -> (w857:string[][])  [unwired: 1 in]
                n488 = Index Array(array=w853, index=0) -> (element=w851:i32)
                n489 = Reshape Array(w857, w851) -> (w850:string[])
                n490 = Search 1D Array(1D array=w850, element="Dielectric (nm):") -> (index of element=w860:i32)  [unwired: 1 in]
                n491 = Equal?(x=w860, y=-1) -> (x = y?=w859:bool)
                n492 = case shown="False" w859 {
                  tunnel: w848 -> [w868 w872]
                  tunnel: w860 -> [w864 _]
                  tunnel: [w863 w872] -> w858
                  frame False {
                    n493 = local read "Rec: Dielectric (d)"() -> (w870:dbl)
                    n494 = Number To Fractional String(number=w870) -> (F-format string=w865:string)  [unwired: 3 in]
                    n495 = Divide(x=w864, y=3) -> (x/y=w867:dbl)
                    n496 = To Word Integer(number=w867) -> (16bit integer=w866:i16)
                    n497 = Replace Array Subset(array=w868, new element=w865, index (row)=w866, index (col)=1) -> (w863:string[][])
                  }
                  frame True {
                  }
                }
                n498 = local write "Save Array"(w858) -> ()
              }
              frame #1 {
                n499 = local read "Save Array"() -> (w874:string[][])
                n500 = Array Size(array=w874) -> (size(s)=w877:i32[])
                n501 = Array Subset(array=w874, index (row)=0, index (col)=0, length (col)=3) -> (w881:string[][])  [unwired: 1 in]
                n502 = Index Array(array=w877, index=0) -> (element=w875:i32)
                n503 = Reshape Array(w881, w875) -> (w873:string[])
                n504 = Search 1D Array(1D array=w873, element="Comments:") -> (index of element=w884:i32)  [unwired: 1 in]
                n505 = Equal?(x=w884, y=-1) -> (x = y?=w883:bool)
                n506 = case shown="False" w883 {
                  tunnel: w874 -> [w892 w895]
                  tunnel: w884 -> [w889 _]
                  tunnel: [w888 w895] -> w882
                  frame False {
                    n507 = local read "New: Comments"() -> (w887:string)
                    n508 = Divide(x=w889, y=3) -> (x/y=w891:dbl)
                    n509 = To Word Integer(number=w891) -> (16bit integer=w890:i16)
                    n510 = Replace Array Subset(array=w892, new element=w887, index (row)=w890, index (col)=1) -> (w888:string[][])
                  }
                  frame True {
                  }
                }
                n511 = local write "Save Array"(w882) -> ()
              }
              frame #2 {
                n512 = local read "Save Array"() -> (w897:string[][])
                n513 = Array Size(array=w897) -> (size(s)=w900:i32[])
                n514 = Array Subset(array=w897, index (row)=0, index (col)=0, length (col)=3) -> (w904:string[][])  [unwired: 1 in]
                n515 = Index Array(array=w900, index=0) -> (element=w898:i32)
                n516 = Reshape Array(w904, w898) -> (w896:string[])
                n517 = Search 1D Array(1D array=w896, element="Length (um):") -> (index of element=w907:i32)  [unwired: 1 in]
                n518 = Equal?(x=w907, y=-1) -> (x = y?=w906:bool)
                n519 = case shown="False" w906 {
                  tunnel: w897 -> [w917 w920]
                  tunnel: w907 -> [w914 _]
                  tunnel: [w913 w920] -> w905
                  frame False {
                    n520 = local read "New: Length"() -> (w910:dbl)
                    n521 = Divide(x=w914, y=3) -> (x/y=w916:dbl)
                    n522 = Format Value(format string="%#g", value (0)=w910) -> (output string=w911:string)  [unwired: 1 in]
                    n523 = To Word Integer(number=w916) -> (16bit integer=w915:i16)
                    n524 = Replace Array Subset(array=w917, new element=w911, index (row)=w915, index (col)=1) -> (w913:string[][])
                  }
                  frame True {
                  }
                }
                n525 = local write "Save Array"(w905) -> ()
              }
              frame #3 {
                n526 = local read "Save Array"() -> (w922:string[][])
                n527 = Array Size(array=w922) -> (size(s)=w927:i32[])
                n528 = Array Subset(array=w922, index (row)=0, index (col)=0, length (col)=3) -> (w923:string[][])  [unwired: 1 in]
                n529 = Index Array(array=w927, index=0) -> (element=w929:i32)
                n530 = Reshape Array(w923, w929) -> (w921:string[])
                n531 = Search 1D Array(1D array=w921, element="Width (um):") -> (index of element=w932:i32)  [unwired: 1 in]
                n532 = Equal?(x=w932, y=-1) -> (x = y?=w931:bool)
                n533 = case shown="False" w931 {
                  tunnel: w932 -> [w940 _]
                  tunnel: w922 -> [w939 w945]
                  tunnel: [w938 w945] -> w930
                  frame False {
                    n534 = local read "New: Width"() -> (w935:dbl)
                    n535 = Divide(x=w940, y=3) -> (x/y=w942:dbl)
                    n536 = To Word Integer(number=w942) -> (16bit integer=w941:i16)
                    n537 = Format Value(format string="%#g", value (0)=w935) -> (output string=w936:string)  [unwired: 1 in]
                    n538 = Replace Array Subset(array=w939, new element=w936, index (row)=w941, index (col)=1) -> (w938:string[][])
                  }
                  frame True {
                  }
                }
                n539 = local write "Save Array"(w930) -> ()
              }
              frame #4 {
                w955 = "Sample Temp (K):"
                n540 = local read "Save Array"() -> (w947:string[][])
                n541 = Array Size(array=w947) -> (size(s)=w952:i32[])
                n542 = Array Subset(array=w947, index (row)=0, index (col)=0, length (col)=3) -> (w948:string[][])  [unwired: 1 in]
                n543 = Index Array(array=w952, index=0) -> (element=w954:i32)
                n544 = Reshape Array(w948, w954) -> (w946:string[])
                n545 = Search 1D Array(1D array=w946, element=w955) -> (index of element=w958:i32)  [unwired: 1 in]
                n546 = Equal?(x=w958, y=-1) -> (x = y?=w957:bool)
                n547 = case shown="True" w957 {
                  tunnel: w947 -> [w967 w981]
                  tunnel: w958 -> [w964 _]
                  tunnel: [w963 w980] -> w956
                  tunnel: w946 -> [_ w983]
                  tunnel: w955 -> [_ w970]
                  frame False {
                    n548 = local read "New: Temp"() -> (w961:dbl)
                    n549 = Divide(x=w964, y=3) -> (x/y=w966:dbl)
                    n550 = Format Value(format string="%#g", value (0)=w961) -> (output string=w960:string)  [unwired: 1 in]
                    n551 = To Word Integer(number=w966) -> (16bit integer=w965:i16)
                    n552 = Replace Array Subset(array=w967, new element=w960, index (row)=w965, index (col)=1) -> (w963:string[][])
                  }
                  frame True {
                    n553 = local read "New: Temp"() -> (w972:dbl)
                    n554 = Search 1D Array(1D array=w983, element="Width (um):") -> (index of element=w977:i32)  [unwired: 1 in]
                    n555 = Divide(x=w977, y=3) -> (x/y=w978:dbl)
                    n556 = To Word Integer(number=w978) -> (16bit integer=w976:i16)
                    n557 = Format Value(format string="%#g", value (0)=w972) -> (output string=w971:string)  [unwired: 1 in]
                    n558 = Build Array(w970, w971) -> (w974:string[])
                    n559 = Increment(x=w976) -> (x+1=w975:i16)
                    n560 = Insert Into Array(array=w981, index (row)=w975, new element=w974) -> (w980:string[][])  [unwired: 1 in]
                  }
                }
                n561 = local write "Save Array"(w956) -> ()
              }
              frame #5 {
                w993 = "Mobility-Sat (cm^2/Vs):"
                n562 = local read "Save Array"() -> (w985:string[][])
                n563 = Array Size(array=w985) -> (size(s)=w990:i32[])
                n564 = Array Subset(array=w985, index (row)=0, index (col)=0, length (col)=3) -> (w986:string[][])  [unwired: 1 in]
                n565 = Index Array(array=w990, index=0) -> (element=w992:i32)
                n566 = Reshape Array(w986, w992) -> (w984:string[])
                n567 = Search 1D Array(1D array=w984, element=w993) -> (index of element=w996:i32)  [unwired: 1 in]
                n568 = Equal?(x=w996, y=-1) -> (x = y?=w995:bool)
                n569 = case shown="True" w995 {
                  tunnel: w985 -> [w1006 w1016]
                  tunnel: w996 -> [w1003 _]
                  tunnel: [w1002 w1015] -> w994
                  tunnel: w984 -> [_ w1013]
                  tunnel: w993 -> [_ w1011]
                  frame False {
                    n570 = local read "Re-Calculated Values Cluster"() -> (w999:T9)
                    n571 = Unbundle By Name(w999) -> ("Mobility-Sat"=w998:dbl)
                    n572 = Divide(x=w1003, y=3) -> (x/y=w1005:dbl)
                    n573 = To Word Integer(number=w1005) -> (16bit integer=w1004:i16)
                    n574 = Format Value(format string="%#g", value (0)=w998) -> (output string=w1000:string)  [unwired: 1 in]
                    n575 = Replace Array Subset(array=w1006, new element=w1000, index (row)=w1004, index (col)=1) -> (w1002:string[][])
                  }
                  frame True {
                    n576 = local read "Re-Calculated Values Cluster"() -> (w1010:T9)
                    n577 = Unbundle By Name(w1010) -> ("Mobility-Sat"=w1009:dbl)
                    n578 = Search 1D Array(1D array=w1013, element="Mobility (cm^2/Vs):") -> (index of element=w1019:i32)  [unwired: 1 in]
                    n579 = Divide(x=w1019, y=3) -> (x/y=w1020:dbl)
                    n580 = To Word Integer(number=w1020) -> (16bit integer=w1012:i16)
                    n581 = Format Value(format string="%#g", value (0)=w1009) -> (output string=w1014:string)  [unwired: 1 in]
                    n582 = Build Array(w1011, w1014) -> (w1018:string[])
                    n583 = Replace Array Subset(array=w1016, new element=w1018, index (row)=w1012) -> (w1015:string[][])  [unwired: 1 in]
                  }
                }
                n584 = local write "Save Array"(w994) -> ()
              }
              frame #6 {
                w1032 = "Mobility-Lin (cm^2/Vs):"
                n585 = local read "Save Array"() -> (w1023:string[][])
                n586 = Array Size(array=w1023) -> (size(s)=w1029:i32[])
                n587 = Array Subset(array=w1023, index (row)=0, index (col)=0, length (col)=3) -> (w1025:string[][])  [unwired: 1 in]
                n588 = Index Array(array=w1029, index=0) -> (element=w1031:i32)
                n589 = Reshape Array(w1025, w1031) -> (w1024:string[])
                n590 = Search 1D Array(1D array=w1024, element=w1032) -> (index of element=w1035:i32)  [unwired: 1 in]
                n591 = Equal?(x=w1035, y=-1) -> (x = y?=w1034:bool)
                n592 = case shown="True" w1034 {
                  tunnel: w1023 -> [w1045 w1053]
                  tunnel: w1035 -> [w1042 _]
                  tunnel: [w1041 w1052] -> w1033
                  tunnel: w1024 -> [_ w1051]
                  tunnel: w1032 -> [_ w1050]
                  frame False {
                    n593 = local read "Re-Calculated Values Cluster"() -> (w1038:T9)
                    n594 = Unbundle By Name(w1038) -> ("Moblitity-Lin"=w1037:dbl)
                    n595 = Divide(x=w1042, y=3) -> (x/y=w1044:dbl)
                    n596 = To Word Integer(number=w1044) -> (16bit integer=w1043:i16)
                    n597 = Format Value(format string="%#g", value (0)=w1037) -> (output string=w1039:string)  [unwired: 1 in]
                    n598 = Replace Array Subset(array=w1045, new element=w1039, index (row)=w1043, index (col)=1) -> (w1041:string[][])
                  }
                  frame True {
                    n599 = local read "Re-Calculated Values Cluster"() -> (w1049:T9)
                    n600 = Unbundle By Name(w1049) -> ("Moblitity-Lin"=w1048:dbl)
                    n601 = Search 1D Array(1D array=w1051, element="Mobility-Sat (cm^2/Vs):") -> (index of element=w1058:i32)  [unwired: 1 in]
                    n602 = Divide(x=w1058, y=3) -> (x/y=w1059:dbl)
                    n603 = To Word Integer(number=w1059) -> (16bit integer=w1057:i16)
                    n604 = Format Value(format string="%#g", value (0)=w1048) -> (output string=w1062:string)  [unwired: 1 in]
                    n605 = Build Array(w1050, w1062) -> (w1055:string[])
                    n606 = Increment(x=w1057) -> (x+1=w1056:i16)
                    n607 = Insert Into Array(array=w1053, index (row)=w1056, new element=w1055) -> (w1052:string[][])  [unwired: 1 in]
                  }
                }
                n608 = local write "Save Array"(w1033) -> ()
              }
              frame #7 {
                w1072 = "On/Off I-Sat:"
                n609 = local read "Save Array"() -> (w1063:string[][])
                n610 = Array Size(array=w1063) -> (size(s)=w1069:i32[])
                n611 = Array Subset(array=w1063, index (row)=0, index (col)=0, length (col)=3) -> (w1065:string[][])  [unwired: 1 in]
                n612 = Index Array(array=w1069, index=0) -> (element=w1071:i32)
                n613 = Reshape Array(w1065, w1071) -> (w1064:string[])
                n614 = Search 1D Array(1D array=w1064, element=w1072) -> (index of element=w1075:i32)  [unwired: 1 in]
                n615 = Equal?(x=w1075, y=-1) -> (x = y?=w1074:bool)
                n616 = case shown="True" w1074 {
                  tunnel: w1063 -> [w1085 w1094]
                  tunnel: w1075 -> [w1082 _]
                  tunnel: [w1081 w1095] -> w1073
                  tunnel: w1064 -> [_ w1092]
                  tunnel: w1072 -> [_ w1090]
                  frame False {
                    n617 = local read "Calculated Values Cluster"() -> (w1078:T9)
                    n618 = Divide(x=w1082, y=3) -> (x/y=w1084:dbl)
                    n619 = Unbundle By Name(w1078) -> ("On/Off"=w1077:dbl)
                    n620 = To Word Integer(number=w1084) -> (16bit integer=w1083:i16)
                    n621 = Format Value(format string="%#g", value (0)=w1077) -> (output string=w1079:string)  [unwired: 1 in]
                    n622 = Replace Array Subset(array=w1085, new element=w1079, index (row)=w1083, index (col)=1) -> (w1081:string[][])
                  }
                  frame True {
                    n623 = local read "Calculated Values Cluster"() -> (w1089:T9)
                    n624 = Unbundle By Name(w1089) -> ("On/Off"=w1088:dbl)
                    n625 = Search 1D Array(1D array=w1092, element="On/Off Current:") -> (index of element=w1098:i32)  [unwired: 1 in]
                    n626 = Divide(x=w1098, y=3) -> (x/y=w1099:dbl)
                    n627 = To Word Integer(number=w1099) -> (16bit integer=w1091:i16)
                    n628 = Format Value(format string="%#g", value (0)=w1088) -> (output string=w1093:string)  [unwired: 1 in]
                    n629 = Build Array(w1090, w1093) -> (w1097:string[])
                    n630 = Replace Array Subset(array=w1094, new element=w1097, index (row)=w1091) -> (w1095:string[][])  [unwired: 1 in]
                  }
                }
                n631 = local write "Save Array"(w1073) -> ()
              }
              frame #8 {
                w1111 = "Off I-Sat (A):"
                n632 = local read "Save Array"() -> (w1102:string[][])
                n633 = Array Size(array=w1102) -> (size(s)=w1108:i32[])
                n634 = Array Subset(array=w1102, index (row)=0, index (col)=0, length (col)=3) -> (w1104:string[][])  [unwired: 1 in]
                n635 = Index Array(array=w1108, index=0) -> (element=w1110:i32)
                n636 = Reshape Array(w1104, w1110) -> (w1103:string[])
                n637 = Search 1D Array(1D array=w1103, element=w1111) -> (index of element=w1114:i32)  [unwired: 1 in]
                n638 = Equal?(x=w1114, y=-1) -> (x = y?=w1113:bool)
                n639 = case shown="True" w1113 {
                  tunnel: w1102 -> [w1124 w1132]
                  tunnel: w1114 -> [w1121 _]
                  tunnel: [w1120 w1131] -> w1112
                  tunnel: w1103 -> [_ w1130]
                  tunnel: w1111 -> [_ w1129]
                  frame False {
                    # "New Data File"
                    n640 = local read "Calculated Values Cluster"() -> (w1117:T9)
                    n641 = Unbundle By Name(w1117) -> ("Off Current"=w1116:dbl)
                    n642 = Divide(x=w1121, y=3) -> (x/y=w1123:dbl)
                    n643 = Format Value(format string="%#g", value (0)=w1116) -> (output string=w1118:string)  [unwired: 1 in]
                    n644 = To Word Integer(number=w1123) -> (16bit integer=w1122:i16)
                    n645 = Replace Array Subset(array=w1124, new element=w1118, index (row)=w1122, index (col)=1) -> (w1120:string[][])
                  }
                  frame True {
                    # "Old Data File"
                    n646 = local read "Calculated Values Cluster"() -> (w1128:T9)
                    n647 = Unbundle By Name(w1128) -> ("Off Current"=w1127:dbl)
                    n648 = Search 1D Array(1D array=w1130, element="On/Off I-Sat:") -> (index of element=w1137:i32)  [unwired: 1 in]
                    n649 = Divide(x=w1137, y=3) -> (x/y=w1138:dbl)
                    n650 = To Word Integer(number=w1138) -> (16bit integer=w1136:i16)
                    n651 = Format Value(format string="%#g", value (0)=w1127) -> (output string=w1141:string)  [unwired: 1 in]
                    n652 = Build Array(w1129, w1141) -> (w1134:string[])
                    n653 = Increment(x=w1136) -> (x+1=w1135:i16)
                    n654 = Insert Into Array(array=w1132, index (row)=w1135, new element=w1134) -> (w1131:string[][])  [unwired: 1 in]
                  }
                }
                n655 = local write "Save Array"(w1112) -> ()
              }
              frame #9 {
                w1143 = "Vt-Sat (V):"
                n656 = local read "Save Array"() -> (w1144:string[][])
                n657 = Array Size(array=w1144) -> (size(s)=w1149:i32[])
                n658 = Array Subset(array=w1144, index (row)=0, index (col)=0, length (col)=3) -> (w1145:string[][])  [unwired: 1 in]
                n659 = Index Array(array=w1149, index=0) -> (element=w1151:i32)
                n660 = Reshape Array(w1145, w1151) -> (w1142:string[])
                n661 = Search 1D Array(1D array=w1142, element=w1143) -> (index of element=w1154:i32)  [unwired: 1 in]
                n662 = Equal?(x=w1154, y=-1) -> (x = y?=w1153:bool)
                n663 = case shown="True" w1153 {
                  tunnel: w1144 -> [w1163 w1173]
                  tunnel: w1154 -> [w1159 _]
                  tunnel: [w1158 w1172] -> w1152
                  tunnel: w1143 -> [_ w1171]
                  tunnel: w1142 -> [_ w1170]
                  frame False {
                    n664 = local read "Re-Calculated Values Cluster"() -> (w1157:T9)
                    n665 = Unbundle By Name(w1157) -> ("Vt-Sat"=w1156:dbl)
                    n666 = Divide(x=w1159, y=3) -> (x/y=w1162:dbl)
                    n667 = To Word Integer(number=w1162) -> (16bit integer=w1161:i16)
                    n668 = Number To Fractional String(number=w1156) -> (F-format string=w1160:string)  [unwired: 3 in]
                    n669 = Replace Array Subset(array=w1163, new element=w1160, index (row)=w1161, index (col)=1) -> (w1158:string[][])
                  }
                  frame True {
                    n670 = local read "Re-Calculated Values Cluster"() -> (w1167:T9)
                    n671 = Unbundle By Name(w1167) -> ("Vt-Sat"=w1166:dbl)
                    n672 = Search 1D Array(1D array=w1170, element="Threshold V (V):") -> (index of element=w1169:i32)  [unwired: 1 in]
                    n673 = Divide(x=w1169, y=3) -> (x/y=w1176:dbl)
                    n674 = To Word Integer(number=w1176) -> (16bit integer=w1168:i16)
                    n675 = Format Value(format string="%#g", value (0)=w1166) -> (output string=w1179:string)  [unwired: 1 in]
                    n676 = Build Array(w1171, w1179) -> (w1175:string[])
                    n677 = Replace Array Subset(array=w1173, new element=w1175, index (row)=w1168) -> (w1172:string[][])  [unwired: 1 in]
                  }
                }
                n678 = local write "Save Array"(w1152) -> ()
              }
              frame #10 {
                n679 = disable-structure shown="Disabled" {
                  frame Disabled {
                    n680 = local read "Save Array"() -> (w1180:string[][])
                    n681 = Array Size(array=w1180) -> (size(s)=w1186:i32[])
                    n682 = Array Subset(array=w1180, index (row)=0, index (col)=0, length (col)=3) -> (w1182:string[][])  [unwired: 1 in]
                    n683 = Index Array(array=w1186, index=0) -> (element=w1188:i32)
                    n684 = Reshape Array(w1182, w1188) -> (w1181:string[])
                    n685 = Search 1D Array(1D array=w1181, element="VT-Lin (V):") -> (index of element=w1191:i32)  [unwired: 1 in]
                    n686 = Equal?(x=w1191, y=-1) -> (x = y?=w1190:bool)
                    n687 = case shown="False" w1190 {
                      tunnel: w1180 -> [w1200 w1203]
                      tunnel: w1191 -> [w1197 _]
                      tunnel: [w1196 w1203] -> w1189
                      frame False {
                        n688 = Divide(x=w1197, y=3) -> (x/y=w1199:dbl)
                        n689 = To Word Integer(number=w1199) -> (16bit integer=w1198:i16)
                        n690 = Format Value(format string="%#g") -> (output string=w1194:string)  [unwired: 2 in]
                        n691 = Replace Array Subset(array=w1200, new element=w1194, index (row)=w1198, index (col)=1) -> (w1196:string[][])
                      }
                      frame True {
                      }
                    }
                    n692 = local write "Save Array"(w1189) -> ()
                  }
                  frame Enabled {
                  }
                }
              }
              frame #11 {
                w1204 = "STS-Sat (V/decade):"
                n693 = local read "Save Array"() -> (w1206:string[][])
                n694 = Array Size(array=w1206) -> (size(s)=w1211:i32[])
                n695 = Array Subset(array=w1206, index (row)=0, index (col)=0, length (col)=3) -> (w1207:string[][])  [unwired: 1 in]
                n696 = Index Array(array=w1211, index=0) -> (element=w1213:i32)
                n697 = Reshape Array(w1207, w1213) -> (w1205:string[])
                n698 = Search 1D Array(1D array=w1205, element=w1204) -> (index of element=w1216:i32)  [unwired: 1 in]
                n699 = Equal?(x=w1216, y=-1) -> (x = y?=w1215:bool)
                n700 = case shown="True" w1215 {
                  tunnel: w1206 -> [w1226 w1234]
                  tunnel: w1216 -> [w1223 _]
                  tunnel: [w1222 w1235] -> w1214
                  tunnel: w1205 -> [_ w1233]
                  tunnel: w1204 -> [_ w1232]
                  frame False {
                    # "Current Data File"
                    n701 = local read "Re-Calculated Values Cluster"() -> (w1218:T9)
                    n702 = Unbundle By Name(w1218) -> ("STS"=w1219:dbl)
                    n703 = Divide(x=w1223, y=3) -> (x/y=w1225:dbl)
                    n704 = To Word Integer(number=w1225) -> (16bit integer=w1224:i16)
                    n705 = Format Value(format string="%#g", value (0)=w1219) -> (output string=w1220:string)  [unwired: 1 in]
                    n706 = Replace Array Subset(array=w1226, new element=w1220, index (row)=w1224, index (col)=1) -> (w1222:string[][])
                  }
                  frame True {
                    # "Old Data File"
                    n707 = local read "Re-Calculated Values Cluster"() -> (w1229:T9)
                    n708 = Unbundle By Name(w1229) -> ("STS"=w1230:dbl)
                    n709 = Search 1D Array(1D array=w1233, element="S.T.S. (V/decade):") -> (index of element=w1238:i32)  [unwired: 1 in]
                    n710 = Divide(x=w1238, y=3) -> (x/y=w1239:dbl)
                    n711 = To Word Integer(number=w1239) -> (16bit integer=w1231:i16)
                    n712 = Format Value(format string="%#g", value (0)=w1230) -> (output string=w1242:string)  [unwired: 1 in]
                    n713 = Build Array(w1232, w1242) -> (w1237:string[])
                    n714 = Replace Array Subset(array=w1234, new element=w1237, index (row)=w1231) -> (w1235:string[][])  [unwired: 1 in]
                  }
                }
                n715 = local write "Save Array"(w1214) -> ()
              }
              frame #12 {
                w1243 = "Trap Density-VT (Traps/Vcm^2):"
                n716 = local read "Save Array"() -> (w1245:string[][])
                n717 = Array Size(array=w1245) -> (size(s)=w1250:i32[])
                n718 = Array Subset(array=w1245, index (row)=0, index (col)=0, length (col)=3) -> (w1246:string[][])  [unwired: 1 in]
                n719 = Index Array(array=w1250, index=0) -> (element=w1252:i32)
                n720 = Reshape Array(w1246, w1252) -> (w1244:string[])
                n721 = Search 1D Array(1D array=w1244, element=w1243) -> (index of element=w1255:i32)  [unwired: 1 in]
                n722 = Equal?(x=w1255, y=-1) -> (x = y?=w1254:bool)
                n723 = case shown="True" w1254 {
                  tunnel: w1245 -> [w1265 w1272]
                  tunnel: w1255 -> [w1261 _]
                  tunnel: [w1260 w1273] -> w1253
                  tunnel: w1244 -> [_ w1271]
                  tunnel: w1243 -> [_ w1270]
                  frame False {
                    n724 = local read "Re-Calculated Values Cluster"() -> (w1258:T9)
                    n725 = Unbundle By Name(w1258) -> ("Trap Density-VT"=w1257:dbl)
                    n726 = Divide(x=w1261, y=3) -> (x/y=w1264:dbl)
                    n727 = To Word Integer(number=w1264) -> (16bit integer=w1263:i16)
                    n728 = Format Value(format string="%#g", value (0)=w1257) -> (output string=w1262:string)  [unwired: 1 in]
                    n729 = Replace Array Subset(array=w1265, new element=w1262, index (row)=w1263, index (col)=1) -> (w1260:string[][])
                  }
                  frame True {
                    n730 = local read "Re-Calculated Values Cluster"() -> (w1269:T9)
                    n731 = Unbundle By Name(w1269) -> ("Trap Density-VT"=w1268:dbl)
                    n732 = Search 1D Array(1D array=w1271, element="STS-Sat (V/decade):") -> (index of element=w1278:i32)  [unwired: 1 in]
                    n733 = Divide(x=w1278, y=3) -> (x/y=w1277:dbl)
                    n734 = To Word Integer(number=w1277) -> (16bit integer=w1279:i16)
                    n735 = Format Value(format string="%#g", value (0)=w1268) -> (output string=w1274:string)  [unwired: 1 in]
                    n736 = Build Array(w1270, w1274) -> (w1281:string[])
                    n737 = Increment(x=w1279) -> (x+1=w1280:i16)
                    n738 = Insert Into Array(array=w1272, index (row)=w1280, new element=w1281) -> (w1273:string[][])  [unwired: 1 in]
                  }
                }
                n739 = local write "Save Array"(w1253) -> ()
              }
              frame #13 {
                w1283 = "Trap Density-STS (Traps/Vcm^2):"
                n740 = local read "Save Array"() -> (w1285:string[][])
                n741 = Array Size(array=w1285) -> (size(s)=w1290:i32[])
                n742 = Array Subset(array=w1285, index (row)=0, index (col)=0, length (col)=3) -> (w1286:string[][])  [unwired: 1 in]
                n743 = Index Array(array=w1290, index=0) -> (element=w1292:i32)
                n744 = Reshape Array(w1286, w1292) -> (w1284:string[])
                n745 = Search 1D Array(1D array=w1284, element=w1283) -> (index of element=w1295:i32)  [unwired: 1 in]
                n746 = Equal?(x=w1295, y=-1) -> (x = y?=w1294:bool)
                n747 = case shown="True" w1294 {
                  tunnel: w1285 -> [w1305 w1312]
                  tunnel: w1295 -> [w1302 _]
                  tunnel: [w1301 w1313] -> w1293
                  tunnel: w1284 -> [_ w1311]
                  tunnel: w1283 -> [_ w1310]
                  frame False {
                    n748 = local read "Re-Calculated Values Cluster"() -> (w1298:T9)
                    n749 = Unbundle By Name(w1298) -> ("Trap Density-STS"=w1297:dbl)
                    n750 = Divide(x=w1302, y=3) -> (x/y=w1304:dbl)
                    n751 = To Word Integer(number=w1304) -> (16bit integer=w1303:i16)
                    n752 = Format Value(format string="%#g", value (0)=w1297) -> (output string=w1299:string)  [unwired: 1 in]
                    n753 = Replace Array Subset(array=w1305, new element=w1299, index (row)=w1303, index (col)=1) -> (w1301:string[][])
                  }
                  frame True {
                    n754 = local read "Re-Calculated Values Cluster"() -> (w1309:T9)
                    n755 = Unbundle By Name(w1309) -> ("Trap Density-STS"=w1308:dbl)
                    n756 = Search 1D Array(1D array=w1311, element="Trap Density-VT (Traps/Vcm^2):") -> (index of element=w1318:i32)  [unwired: 1 in]
                    n757 = Divide(x=w1318, y=3) -> (x/y=w1319:dbl)
                    n758 = To Word Integer(number=w1319) -> (16bit integer=w1317:i16)
                    n759 = Format Value(format string="%#g", value (0)=w1308) -> (output string=w1322:string)  [unwired: 1 in]
                    n760 = Build Array(w1310, w1322) -> (w1315:string[])
                    n761 = Increment(x=w1317) -> (x+1=w1316:i16)
                    n762 = Insert Into Array(array=w1312, index (row)=w1316, new element=w1315) -> (w1313:string[][])  [unwired: 1 in]
                  }
                }
                n763 = local write "Save Array"(w1293) -> ()
              }
            }
            n764 = local read "New: Temp"() -> (w830:dbl)
            n765 = local read "New: Width"() -> (w831:dbl)
            n766 = local read "New: Length"() -> (w833:dbl)
            n767 = local read "Index"() -> (w832:string)
            n768 = To Single Precision Float(number=w830) -> (single precision float=w847:sgl)
            n769 = Number To Decimal String(number=w847) -> (decimal integer string=w842:string)  [unwired: 1 in]
            n770 = To Single Precision Float(number=w831) -> (single precision float=w846:sgl)
            n771 = To Single Precision Float(number=w833) -> (single precision float=w845:sgl)
            n772 = Strip Path(path=w829) -> (stripped path=w834:path)  [unwired: 1 out]
            n773 = Number To Decimal String(number=w845) -> (decimal integer string=w840:string)  [unwired: 1 in]
            n774 = Number To Decimal String(number=w846) -> (decimal integer string=w839:string)  [unwired: 1 in]
            n775 = Concatenate Strings("_", w842, "K") -> (w844:string)
            n776 = call "Build Text"("Temp"=w844, "Index"=w832, "Length"=w840, "Width"=w839) -> ("Result"=w838:string)  [unwired: 10 in, 1 out]
            n777 = Path To String(path=w834) -> (string=w836:string)
            n778 = Concatenate Strings(w836, "\\", w838) -> (w837:string)
            n779 = String To Path(string=w837) -> (path=w828:path)
          }
          frame #1 {
            n780 = flat-sequence {
              tunnel: w1326 -> [w1328]
              tunnel: w1325 -> [w1327]
              tunnel: [w1327] -> w1324
              tunnel: w1324 -> [w1334]
              tunnel: w1323 -> [w1333]
              frame #0 {
                n781 = Equal?(x=w1328, y=w1327) -> (x = y?=w1329:bool)
                n782 = case shown="False" w1329 {
                  tunnel: w1328 -> [w1332 _]
                  tunnel: w1327 -> [w1331 _]
                  frame False {
                    n783 = Move(source path=w1332, 9:TRUE, 10:w1331) -> ()  [unwired: 2 in, 3 out]
                  }
                  frame True {
                  }
                }
              }
              frame #1 {
                n784 = local write "Transfer File"(w1334) -> ()
                n785 = call-poly <vilib>:"Write To Spreadsheet File.vi"("2D data"=w1333, "file path (dialog if empty)"=w1334) -> ()  [unwired: 6 in, 1 out]
              }
            }
          }
        }
        n786 = local read "Save Next?"() -> (w814:bool)
        n787 = Cluster To Array(cluster=w819) -> (array=w818:bool[])
        n788 = Boolean Array To Number(Boolean array=w818) -> (number=w817:u32)
        n789 = Equal To 0?(x=w817) -> (x = 0?=w816:bool)
        n790 = case shown="True" w816 {
          tunnel: [MegaAwesome_States."Read Data" w826] -> w815
          tunnel: w814 -> [_ w823]
          frame False {
          }
          frame True {
            n791 = Select(t=MegaAwesome_States."Next File", s=w823, f=MegaAwesome_States."No Event") -> (s? t:f=w826:T2)
          }
        }
      }
      frame "Exit" {
        n792 = disable-structure shown="Disabled" {
          disable-tunnel: [w1338 _] -> _
          disable-tunnel: [w1337 _] -> _
          frame Disabled {
            n793 = flat-sequence {
              tunnel: [w1347] -> w1338
              tunnel: [w1347] -> w1337
              frame #0 {
                w1346 = FALSE
                n794 = property on="Next File" class="Bool (strict)"("Value"=w1346) -> (error out=w1341:errorcluster)  [unwired: 2 in, 1 out]
                n795 = property on="Previous File" class="Bool (strict)"(error in=w1341, "Value"=w1346) -> (error out=w1342:errorcluster)  [unwired: 1 in, 1 out]
                n796 = Request Deallocation(TRUE) -> ()
                n797 = property on="Save" class="Bool (strict)"(error in=w1342, "Value"=w1346) -> (error out=w1343:errorcluster)  [unwired: 1 in, 1 out]
                n798 = property on="Export" class="Bool (strict)"("Value"=w1346) -> ()  [unwired: 2 in, 2 out]
                n799 = property on="Save Next" class="Bool (strict)"(error in=w1343, "Value"=w1346) -> (error out=w1344:errorcluster)  [unwired: 1 in, 1 out]
                n800 = property on="Discard" class="Bool (strict)"(error in=w1344, "Value"=w1346) -> (error out=w1345:errorcluster)  [unwired: 1 in, 1 out]
                n801 = property on="Save Lines" class="Bool (strict)"(error in=w1345, "Value"=w1346) -> ()  [unwired: 1 in, 2 out]
                n802 = property on="Close" class="Bool (strict)"("Value"=w1346) -> ()  [unwired: 2 in, 2 out]
                n803 = property on="Disable Flag" class="Bool (strict)"("Value"=w1346) -> ()  [unwired: 2 in, 2 out]
                n804 = call "IMAQ Dispose"("All Images? (No)"=TRUE) -> ()  [unwired: 5 in, 1 out]
              }
              frame #1 {
                w1347 = MegaAwesome_States."Exit"
              }
            }
          }
          frame Enabled {
          }
        }
        n805 = event shown="[0] Application Instance Close?" {
          selector: _ -> [_]
          dyn-events: _ -> [_]
          timeout: _ -> [_]
          event Application Instance Close? {
            n806 = event-data() -> ()  [unwired: 1 in, 4 out]
            n807 = event-data("Discard?"=TRUE) -> ()  [unwired: 2 in, 1 out]
          }
        }
      }
      frame "Save Lines" {
        n808 = Build Path(base path=w1350, name or relative path="ROI") -> (appended path=w1353:path)
        n809 = call <vilib>:"Check if File or Folder Exists.vi"("path"=w1353) -> ("file or folder exists?"=w1351:bool, "dup path"=w1354:path)  [unwired: 8 in, 1 out]
        n810 = case shown="False" w1351 {
          tunnel: w1354 -> [w1362 w1363]
          tunnel: [w1361 w1363] -> w1358
          frame False {
            n811 = Create Folder(path (use dialog)=w1362) -> (created path=w1361:path)  [unwired: 2 in, 2 out]
          }
          frame True {
          }
        }
        n812 = local read "Index"() -> (w1349:string)
        n813 = property on="Image Out" class="ImageControl"() -> ("ROI"=w1355:T17)  [unwired: 2 in, 2 out]
        n814 = Build Path(base path=w1358, name or relative path=w1349) -> (appended path=w1357:path)
        n815 = Flatten To String(anything=w1355) -> (data string=w1356:string)  [unwired: 3 in, 2 out]
        n816 = Write to Text File(file (use dialog)=w1357, text=w1356) -> ()  [unwired: 2 in, 3 out]
      }
      frame "Export" {
        n817 = flat-sequence {
          tunnel: ["Independant Variable:"] -> w1364
          tunnel: w1365 -> [w1421]
          tunnel: w1364 -> [w1420]
          frame #0 {
            n818 = stacked-sequence {
              tunnel: "Independant Variable:" -> [w1369 w1374 w1379 w1384 w1389 w1394 w1399 w1404 w1409 w1414]
              frame #0 {
                n819 = Equal?(x=w1369, y="Length (um):") -> (x = y?=w1370:bool)
                n820 = case shown="True" w1370 {
                  frame False {
                  }
                  frame True {
                    n821 = local write "X Axis Display Type"("1") -> ()
                    n822 = local write "Opj X Axis"("2") -> ()
                  }
                }
              }
              frame #1 {
                n823 = Equal?(x=w1374, y="Sample Temp (K):") -> (x = y?=w1375:bool)
                n824 = case shown="True" w1375 {
                  frame False {
                  }
                  frame True {
                    n825 = local write "X Axis Display Type"("1") -> ()
                    n826 = local write "Opj X Axis"("1") -> ()
                  }
                }
              }
              frame #2 {
                n827 = Equal?(x=w1379, y="Mobility-Sat (cm^2/Vs):") -> (x = y?=w1380:bool)
                n828 = case shown="True" w1380 {
                  frame False {
                  }
                  frame True {
                    n829 = local write "X Axis Display Type"("2") -> ()
                    n830 = local write "Opj X Axis"("2") -> ()
                  }
                }
              }
              frame #3 {
                n831 = Equal?(x=w1384, y="Mobility-Lin (cm^2/Vs):") -> (x = y?=w1385:bool)
                n832 = case shown="True" w1385 {
                  frame False {
                  }
                  frame True {
                    n833 = local write "X Axis Display Type"("2") -> ()
                    n834 = local write "Opj X Axis"("2") -> ()
                  }
                }
              }
              frame #4 {
                n835 = Equal?(x=w1389, y="On/Off I-Sat:") -> (x = y?=w1390:bool)
                n836 = case shown="True" w1390 {
                  frame False {
                  }
                  frame True {
                    n837 = local write "X Axis Display Type"("2") -> ()
                    n838 = local write "Opj X Axis"("2") -> ()
                  }
                }
              }
              frame #5 {
                n839 = Equal?(x=w1394, y="Off I-Sat (A):") -> (x = y?=w1395:bool)
                n840 = case shown="True" w1395 {
                  frame False {
                  }
                  frame True {
                    n841 = local write "X Axis Display Type"("2") -> ()
                    n842 = local write "Opj X Axis"("2") -> ()
                  }
                }
              }
              frame #6 {
                n843 = Equal?(x=w1399, y="Vt-Sat (V):") -> (x = y?=w1400:bool)
                n844 = case shown="True" w1400 {
                  frame False {
                  }
                  frame True {
                    n845 = local write "X Axis Display Type"("1") -> ()
                    n846 = local write "Opj X Axis"("1") -> ()
                  }
                }
              }
              frame #7 {
                n847 = Equal?(x=w1404, y="STS-Sat (V/decade):") -> (x = y?=w1405:bool)
                n848 = case shown="True" w1405 {
                  frame False {
                  }
                  frame True {
                    n849 = local write "X Axis Display Type"("1") -> ()
                    n850 = local write "Opj X Axis"("1") -> ()
                  }
                }
              }
              frame #8 {
                n851 = Equal?(x=w1409, y="Trap Density-VT (Traps/Vcm^2):") -> (x = y?=w1410:bool)
                n852 = case shown="True" w1410 {
                  frame False {
                  }
                  frame True {
                    n853 = local write "X Axis Display Type"("2") -> ()
                    n854 = local write "Opj X Axis"("2") -> ()
                  }
                }
              }
              frame #9 {
                n855 = Equal?(x=w1414, y="Trap Density-STS (Traps/Vcm^2):") -> (x = y?=w1415:bool)
                n856 = case shown="True" w1415 {
                  frame False {
                  }
                  frame True {
                    n857 = local write "X Axis Display Type"("2") -> ()
                    n858 = local write "Opj X Axis"("2") -> ()
                  }
                }
              }
            }
          }
          frame #1 {
            n859 = local read "Transfer Folder"() -> (w1425:path)
            n860 = Build Path(base path=w1425, name or relative path="Stats") -> (appended path=w1426:path)
            n861 = call <vilib>:"Check if File or Folder Exists.vi"("path"=w1426) -> ("file or folder exists?"=w1440:bool, "dup path"=w1439:path)  [unwired: 8 in, 1 out]
            n862 = call <userlib>:"OA_ConnectToOrigin.vi"() -> ("error out"=w1437:errorcluster, "Origin.IOApplication"=w1438:refnum<k7>)  [unwired: 8 in]
            n863 = case shown="False" w1440 {
              tunnel: w1439 -> [w1613 w1614]
              tunnel: [w1612 w1614] -> w1424
              frame False {
                n864 = Create Folder(path (use dialog)=w1613) -> (created path=w1612:path)  [unwired: 2 in, 2 out]
              }
              frame True {
              }
            }
            n865 = call "File Dialog"("start path"=w1426) -> ("selected path"=w1428:path)  [unwired: 11 in, 3 out]
            n866 = call <userlib>:"OA_Load.vi"("error in (no error)"=w1437, "Path"=w1421, "Origin.IOApplication"=w1438) -> ("error out"=w1435:errorcluster, "Origin.IOApplication"=w1436:refnum<k7>)  [unwired: 1 out]
            n867 = call "OAExecute.vi"("script"="document -m 3;", "Error IO"=w1435, "Origin.IOApplication"=w1436) -> ("Error IO Out"=w1433:errorcluster, "Origin.IOApplication"=w1434:refnum<k7>)  [unwired: 1 in, 1 out]
            n868 = stacked-sequence {
              tunnel: w1425 -> [w1451 w1481 w1493 w1515 w1535 w1556 w1577 w1600]
              tunnel: w1424 -> [w1452 w1480 w1494 w1514 w1536 w1557 w1578 w1601]
              tunnel: w1434 -> [w1454 w1478 w1496 w1517 w1538 w1559 w1580 w1603]
              tunnel: w1433 -> [w1453 w1479 w1495 w1516 w1537 w1558 w1579 w1602]
              tunnel: [_ _ _ _ _ _ _ w1598] -> w1423
              tunnel: [_ _ _ _ _ _ _ w1599] -> w1422
              tunnel: w1420 -> [w1450 w1471 w1492 w1513 w1534 w1555 w1576 w1597]
              frame #0 {
                n869 = local read "X Axis Display Type"() -> (w1442:string)
                n870 = local read "Opj X Axis"() -> (w1447:string)
                n871 = Concatenate Strings("window -a MOBLGraph;\nlayer.x.type=", w1447, "; layer.x.label.numFormat = ", w1442, "; Y3 = 1; X3 = 1;", "window -a MOBLTable;\nwindow -s TV;") -> (w1445:string)
                n872 = call "Param_Analysis_7_24b_JW.vi"("Independant Variable"=w1450, "error in (no error)"=w1453, "Data Folder"=w1451, "Parameter String"="Mobility-Lin (cm^2/Vs):", "Parameter Name"="Mobility-Lin", "Stats Folder"=w1452) -> ("error out"=w1456:errorcluster, "Output Array"=w1458:string[][], "Variables"=w1449:T27)  [unwired: 2 in, 1 out]
                n873 = call "Origin_Export_7_27a_JW.vi"("Input Conditions"=w1449, "Analysis Array"=w1458, "error in (no error)"=w1456, "Parameter Worksheet Name"="[MOBLTable]Mobilities", "Parameter Folder Script"="pe_cd \"Mobility-Lin\";", "Origin.IOApplication"=w1454) -> ("error out"=w1455:errorcluster, "reference out"=w1457:refnum<k7>)  [unwired: 3 in, 1 out]
                n874 = call "OAExecute.vi"("script"=w1445, "Error IO"=w1455, "Origin.IOApplication"=w1457) -> ()  [unwired: 1 in, 3 out]
              }
              frame #1 {
                n875 = local read "X Axis Display Type"() -> (w1463:string)
                n876 = local read "Opj X Axis"() -> (w1468:string)
                n877 = Concatenate Strings("window -a MOBSGraph;\nlayer.x.type=", w1468, "; layer.x.label.numFormat = ", w1463, "; Y3 = 1; X3 = 1;", "window -a MOBSTable;\nwindow -s TV;") -> (w1466:string)
                n878 = call "Param_Analysis_7_24b_JW.vi"("Independant Variable"=w1471, "error in (no error)"=w1479, "Data Folder"=w1481, "Parameter String"="Mobility-Sat (cm^2/Vs):", "Parameter Name"="Mobility-Sat", "Stats Folder"=w1480) -> ("error out"=w1474:errorcluster, "Output Array"=w1472:string[][], "Variables"=w1470:T27)  [unwired: 2 in, 1 out]
                n879 = call "Origin_Export_7_27a_JW.vi"("Input Conditions"=w1470, "Analysis Array"=w1472, "error in (no error)"=w1474, "Parameter Worksheet Name"="[MOBSTable]Mobilities", "Parameter Folder Script"="pe_cd \"Mobility-Sat\";", "Origin.IOApplication"=w1478) -> ("error out"=w1473:errorcluster, "reference out"=w1475:refnum<k7>)  [unwired: 3 in, 1 out]
                n880 = call "OAExecute.vi"("script"=w1466, "Error IO"=w1473, "Origin.IOApplication"=w1475) -> ()  [unwired: 1 in, 3 out]
              }
              frame #2 {
                n881 = local read "X Axis Display Type"() -> (w1484:string)
                n882 = local read "Opj X Axis"() -> (w1489:string)
                n883 = Concatenate Strings("window -a NSTSGraph;\nlayer.x.type=", w1489, "; layer.x.label.numFormat = ", w1484, "; Y3 = 1; X3 = 1;", "window -a NSTSTable;\nwindow -s TV;") -> (w1487:string)
                n884 = call "Param_Analysis_7_24b_JW.vi"("Independant Variable"=w1492, "error in (no error)"=w1495, "Data Folder"=w1493, "Parameter String"="Trap Density-STS (Traps/Vcm^2):", "Parameter Name"="Trap Density-STS", "Stats Folder"=w1494) -> ("error out"=w1499:errorcluster, "Output Array"=w1497:string[][], "Variables"=w1491:T27)  [unwired: 2 in, 1 out]
                n885 = call "Origin_Export_7_27a_JW.vi"("Input Conditions"=w1491, "Analysis Array"=w1497, "error in (no error)"=w1499, "Parameter Worksheet Name"="[NSTSTable]Trap Densities", "Parameter Folder Script"="pe_cd \"N-STS\";", "Origin.IOApplication"=w1496) -> ("error out"=w1498:errorcluster, "reference out"=w1500:refnum<k7>)  [unwired: 3 in, 1 out]
                n886 = call "OAExecute.vi"("script"=w1487, "Error IO"=w1498, "Origin.IOApplication"=w1500) -> ()  [unwired: 1 in, 3 out]
              }
              frame #3 {
                n887 = local read "X Axis Display Type"() -> (w1505:string)
                n888 = local read "Opj X Axis"() -> (w1510:string)
                n889 = call "Param_Analysis_7_24b_JW.vi"("Independant Variable"=w1513, "error in (no error)"=w1516, "Data Folder"=w1515, "Parameter String"="Trap Density-VT (Traps/Vcm^2):", "Parameter Name"="Trap Density-Vt", "Stats Folder"=w1514) -> ("error out"=w1520:errorcluster, "Output Array"=w1518:string[][], "Variables"=w1512:T27)  [unwired: 2 in, 1 out]
                n890 = Concatenate Strings("window -a NVtGraph;\nlayer.x.type=", w1510, "; layer.x.label.numFormat = ", w1505, "; Y3 = 1; X3 = 1;", "window -a NVtTable;\nwindow -s TV;") -> (w1508:string)
                n891 = call "Origin_Export_7_27a_JW.vi"("Input Conditions"=w1512, "Analysis Array"=w1518, "error in (no error)"=w1520, "Parameter Worksheet Name"="[NVTTable]Trap Densities", "Parameter Folder Script"="pe_cd \"N-Vt\";", "Origin.IOApplication"=w1517) -> ("error out"=w1519:errorcluster, "reference out"=w1521:refnum<k7>)  [unwired: 3 in, 1 out]
                n892 = call "OAExecute.vi"("script"=w1508, "Error IO"=w1519, "Origin.IOApplication"=w1521) -> ()  [unwired: 1 in, 3 out]
              }
              frame #4 {
                n893 = local read "X Axis Display Type"() -> (w1526:string)
                n894 = local read "Opj X Axis"() -> (w1531:string)
                n895 = Concatenate Strings("window -a OffIGraph;\nlayer.x.type=", w1531, "; layer.x.label.numFormat = ", w1526, "; Y3 = 1; X3 = 1;", "window -a OffITable;\nwindow -s TV;") -> (w1529:string)
                n896 = call "Param_Analysis_7_24b_JW.vi"("Independant Variable"=w1534, "error in (no error)"=w1537, "Data Folder"=w1535, "Parameter String"="Off I-Sat (A):", "Parameter Name"="Off I-Sat", "Stats Folder"=w1536) -> ("error out"=w1541:errorcluster, "Output Array"=w1539:string[][], "Variables"=w1533:T27)  [unwired: 2 in, 1 out]
                n897 = call "Origin_Export_7_27a_JW.vi"("Input Conditions"=w1533, "Analysis Array"=w1539, "error in (no error)"=w1541, "Parameter Worksheet Name"="[OffItable]OffCurrents", "Parameter Folder Script"="pe_cd \"OffI-Sat\";", "Origin.IOApplication"=w1538) -> ("error out"=w1540:errorcluster, "reference out"=w1542:refnum<k7>)  [unwired: 3 in, 1 out]
                n898 = call "OAExecute.vi"("script"=w1529, "Error IO"=w1540, "Origin.IOApplication"=w1542) -> ()  [unwired: 1 in, 3 out]
              }
              frame #5 {
                n899 = local read "X Axis Display Type"() -> (w1547:string)
                n900 = local read "Opj X Axis"() -> (w1552:string)
                n901 = Concatenate Strings("window -a OnOffGraph;\nlayer.x.type=", w1552, "; layer.x.label.numFormat = ", w1547, "; Y3 = 1; X3 = 1;", "window -a OnOffTable;\nwindow -s TV;") -> (w1550:string)
                n902 = call "Param_Analysis_7_24b_JW.vi"("Independant Variable"=w1555, "error in (no error)"=w1558, "Data Folder"=w1556, "Parameter String"="On/Off I-Sat:", "Parameter Name"="OnOff Ratio", "Stats Folder"=w1557) -> ("error out"=w1562:errorcluster, "Output Array"=w1560:string[][], "Variables"=w1554:T27)  [unwired: 2 in, 1 out]
                n903 = call "Origin_Export_7_27a_JW.vi"("Input Conditions"=w1554, "Analysis Array"=w1560, "error in (no error)"=w1562, "Parameter Worksheet Name"="[OnOffTable]On/Off Ratios", "Parameter Folder Script"="pe_cd \"OnOff-Ratio\";", "Origin.IOApplication"=w1559) -> ("error out"=w1561:errorcluster, "reference out"=w1563:refnum<k7>)  [unwired: 3 in, 1 out]
                n904 = call "OAExecute.vi"("script"=w1550, "Error IO"=w1561, "Origin.IOApplication"=w1563) -> ()  [unwired: 1 in, 3 out]
              }
              frame #6 {
                n905 = local read "X Axis Display Type"() -> (w1568:string)
                n906 = local read "Opj X Axis"() -> (w1573:string)
                n907 = call "Param_Analysis_7_24b_JW.vi"("Independant Variable"=w1576, "error in (no error)"=w1579, "Data Folder"=w1577, "Parameter String"="STS-Sat (V/decade):", "Parameter Name"="STS-Sat", "Stats Folder"=w1578) -> ("error out"=w1583:errorcluster, "Output Array"=w1581:string[][], "Variables"=w1575:T27)  [unwired: 2 in, 1 out]
                n908 = Concatenate Strings("window -a SGraph;\nlayer.x.type=", w1573, "; layer.x.label.numFormat = ", w1568, "; Y3 = 1; X3 = 1;", "window -a STable;\nwindow -s TV;") -> (w1571:string)
                n909 = call "Origin_Export_7_27a_JW.vi"("Input Conditions"=w1575, "Analysis Array"=w1581, "error in (no error)"=w1583, "Parameter Worksheet Name"="[STable]Threshold Swing", "Parameter Folder Script"="pe_cd \"STS-Sat\";", "Origin.IOApplication"=w1580) -> ("error out"=w1582:errorcluster, "reference out"=w1584:refnum<k7>)  [unwired: 3 in, 1 out]
                n910 = call "OAExecute.vi"("script"=w1571, "Error IO"=w1582, "Origin.IOApplication"=w1584) -> ()  [unwired: 1 in, 3 out]
              }
              frame #7 {
                n911 = local read "X Axis Display Type"() -> (w1589:string)
                n912 = local read "Opj X Axis"() -> (w1594:string)
                n913 = Concatenate Strings("window -a VtGraph;\nlayer.x.type=", w1594, "; layer.x.label.numFormat = ", w1589, "; Y3 = 1; X3 = 1;", "window -a VtTable;\nwindow -s TV;") -> (w1592:string)
                n914 = call "Param_Analysis_7_24b_JW.vi"("Independant Variable"=w1597, "error in (no error)"=w1602, "Data Folder"=w1600, "Parameter String"="Vt-Sat (V):", "Parameter Name"="Vt-Sat", "Stats Folder"=w1601) -> ("error out"=w1606:errorcluster, "Output Array"=w1604:string[][], "Variables"=w1596:T27)  [unwired: 2 in, 1 out]
                n915 = call "Origin_Export_7_27a_JW.vi"("Input Conditions"=w1596, "Analysis Array"=w1604, "error in (no error)"=w1606, "Parameter Worksheet Name"="[VtTable]Threshold Voltages", "Parameter Folder Script"="pe_cd \"Vt-Sat\";", "Origin.IOApplication"=w1603) -> ("error out"=w1605:errorcluster, "reference out"=w1607:refnum<k7>)  [unwired: 3 in, 1 out]
                n916 = call "OAExecute.vi"("script"=w1592, "Error IO"=w1605, "Origin.IOApplication"=w1607) -> ("Error IO Out"=w1598:errorcluster, "Origin.IOApplication"=w1599:refnum<k7>)  [unwired: 1 in, 1 out]
              }
            }
            n917 = Path To String(path=w1428) -> (string=w1427:string)
            n918 = call "OAExecute.vi"("script"="pe_cd /; ", "Error IO"=w1423, "Origin.IOApplication"=w1422) -> ("Error IO Out"=w1429:errorcluster, "Origin.IOApplication"=w1430:refnum<k7>)  [unwired: 1 in, 1 out]
            n919 = call <userlib>:"OASaveProject.vi"("path"=w1427, "Error IO"=w1429, "Origin.IOApplication"=w1430) -> ("Origin.IOApplication"=w1419:refnum<k7>)  [unwired: 2 out]
            n920 = call <userlib>:"OAEndSession.vi"("Origin.IOApplication"=w1419) -> ()  [unwired: 1 in, 3 out]
          }
        }
      }
    }
    "Current State" <- w11
    "Folder Index" <- w21
    n921 = Wait (ms)(milliseconds to wait=u32 50) -> ()  [unwired: 1 out]
    n922 = Equal?(x=w11, y=MegaAwesome_States."Exit") -> (x = y?=w14:bool)
  }
  n923 = disable-structure shown="Disabled" {
    disable-tunnel: w1 -> [w1616 _]
    frame Disabled {
      n924 = call "Close LabView?"("Enable"=w1616) -> ("OK"=w1615:bool)  [unwired: 17 in, 1 out]
      n925 = Quit LabVIEW(quit? (T)=w1615) -> ()
    }
    frame Enabled {
    }
  }
